vi "Main FTS.vi"() -> ()   [LabVIEW 2015]
uses:
  Controls/Gen2 FT states.ctl
  SubVI/ESTOP CONTROL.ctl
  Controls/Target RF Channel.ctl
  Controls/InfoPacket.ctl
  Controls/FTS Main Current Channel.ctl
  <vilib>/Utility/error.llb/DialogType.ctl
  Controls/LocalVars.ctl
  Controls/Iniial Device Programming.ctl
  SubVI/ProgramStageControl.ctl
  Controls/Batt Cap Steps.ctl
  Controls/Support Script.ctl
  Controls/Serial Table.ctl
  Controls/Device Information.ctl
  Controls/Loading.ctl
  Controls/Load Step.ctl
  Controls/Mark10 Config.ctl
  Controls/PID parameters.ctl
  Controls/Channels.ctl
  RxTx/XceiverStates.ctl
  Controls/Mark10 states.ctl
  RxTx/XceiverCmds.ctl
  Controls/Gen2 FT Globals.vi
  <vilib>/Utility/config.llb/Write Key (I32).vi
  <vilib>/Utility/config.llb/Write Key (String).vi
  <vilib>/Utility/config.llb/NI_LVConfig.lvlib
panel:
  out "Prog Page #":i32
  out "Time:":timestamp
  out "Transceiver Channel":u8 caption="Start Channel"
  in  "Start Channel":T1="5"
  out "Main":i32
  out "Read":i32
  in  "Correction Factor":string caption="Correction Factor:"
  out "Current Time:":timestamp=timestamp(3438190648.7035365 s since 1904-01-01) format="%<%I:%M:%S %p\n%m/%d/%Y>T"
  in  "Tab Control":T2(tab)
  in  "Eng Log?":bool
  in  "Blast Shutdown":bool=TRUE
  in  "Home":bool
  in  "GotoPosition":bool
  in  "GotoLoad":bool
  in  "Position(inch)":dbl format="%.2f"
  in  "Load(lbs):":dbl format="%.2g"
  in  "MoveUp":bool
  in  "MoveDown":bool
  in  "StopMotor":bool
  out "Gauge Load":dbl format="%.2f"
  out "Gauge Position":dbl format="%.3f"
  out "RawData":u16[](array[numeric]) caption="RawData\n      S2           S3             S4           S5           S6           S7          Ref1       Ref2        Batt"
  out "Adj.Data":dbl[](array[numeric])
  out "Front Panel Data":dbl[][](array[numeric]) format="%.2f"
  in  "Mark-10 COM Port":refnum<visa-resource-name>="COM1"
  in  "Override 4th Test":bool=TRUE
  in  "Reset Device":bool=TRUE
  out "Device Parameters":T3 {"ASICtrim" format="%02x"}
  out "GotCal":bool
  out "Streaming Serial Number":u32
  in  "Refresh Button":bool
  in  "Change Path":bool
  out "Serial Folder Path":path
  out "Serial Table Lookup":string[][](array[string]) caption="Serial Number               Lot Number            Brand Prefix              Type                        Device ID"
  in  "Close Xsceiver":bool
  in  "Scan Channels":bool
  in  "Clear Messages":bool caption="DevOFF"
  out "Test Result":bool
  in  "Operator":string caption="Operator Name:"
  in  "Target Channel":T4="5"
  in  "Operating Channel":string(combo)="5"
  out "Rev String":string
  out "Device Image":picture
  out "Battery Voltage":dbl format="%.2g"
  out "Accelerometer sample size":i32
  out "Base Accels":dbl[][](array[numeric])
  out "Six Plane Accels":dbl[][](array[numeric])
  in  "CaptureButton":bool
  out "Message":string
  out "AssemScore":i32
  out "PCB Score":i32
  out "Three Failed Tests":dbl
  out "Unit failed 3x Tests":bool
  in  "Target Serial#:":u32 caption="Serial#:" max=268435455
  out "Brand:":string
  out "DeviceType:":string
  out "Device ON?":bool
  in  "Test Device":bool
  out "SoftwareVersion":string="SW-03004-000\nRevision 1.0"
  out "DeviceID:":string
  out "Lot#:":string
  in  "ClearBuffer":bool
  in  "Exit":bool
  in  "Estop":T5
  in  "Shutdown Dev":bool caption="DevOFF"
  in  "States":T6=enum."Initialization"
  out "error out":errorcluster
  # "©2013 Aztera LLC"
  # "OrthoSensor Device Calibration"
  # "System Messages"
  # "Device"
  # "Device Information"
  # "Required Inputs"
  # "lbs"
  # "inch"
  # "Mark-10"
  # "Target Loads\n(lbs)"
  # "Gauge Loads\n(lbs)"
  # "Total Device \nLoads (lbs)"
  # "Device Loads"
  # "Errors"
  # "A (lbs)            B (lbs)"
  # "A (lbs)            B (lbs)"
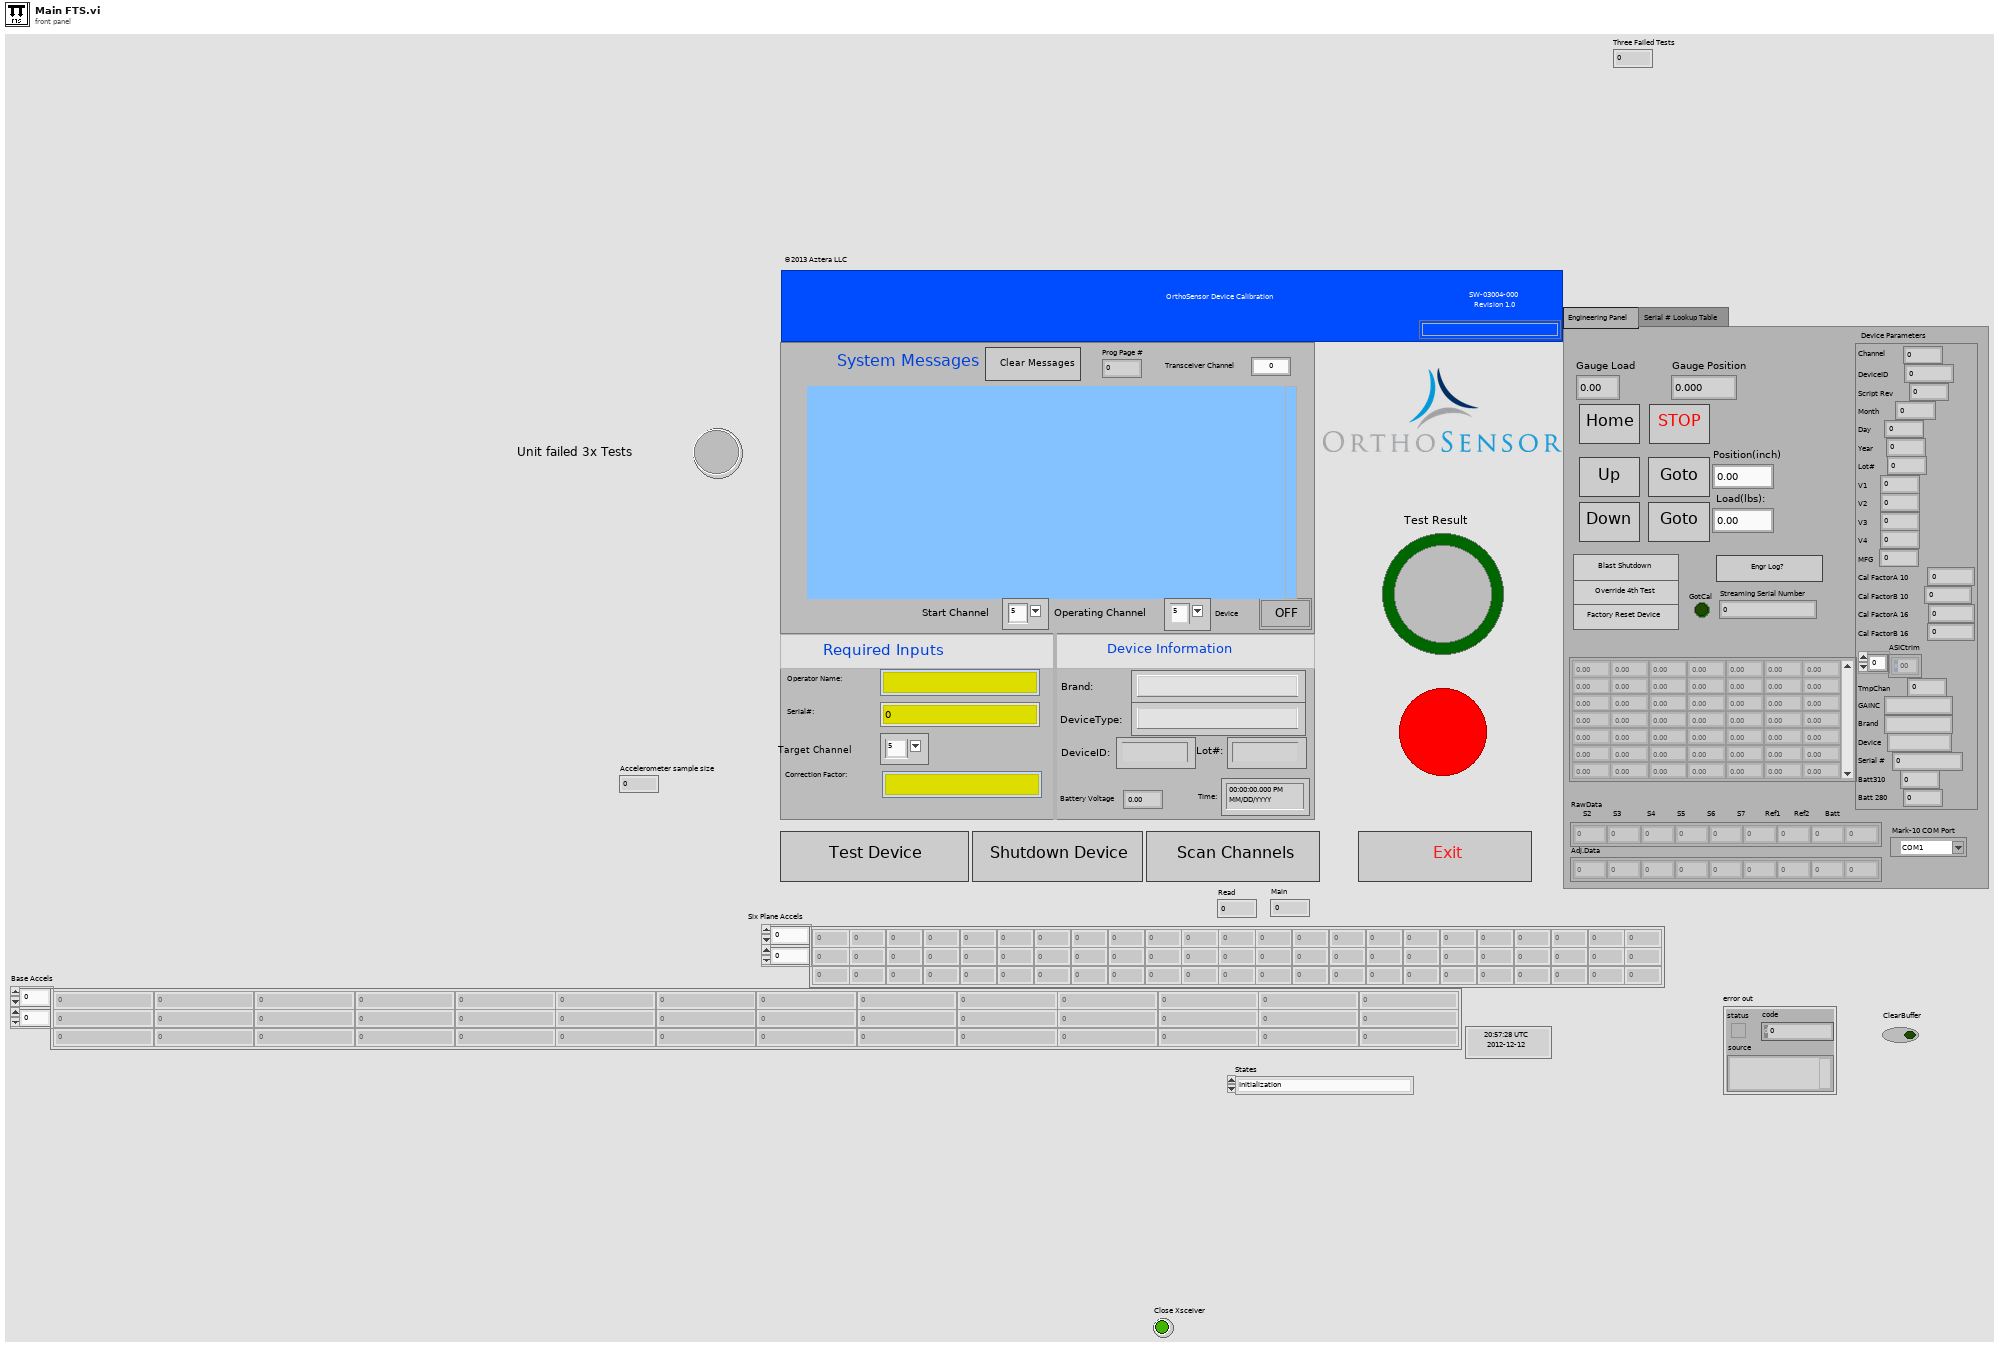
[diagram p1: front panel]
types:
  T1 = typedef "FTS Main Current Channel.ctl" = string
  T2 = enum32{"Engineering Panel", "Serial # Lookup Table"}
  T3 = typedef "InfoPacket.ctl" = cluster{"Channel":u8, "DeviceID":u32, "Script Rev":u8, "Month":u8, "Day":u8, "Year":u8, "Lot#":u32, "V1":u16, "V2":u16, "V3":u16, "V4":u16, "MFG":u8, "Cal FactorA 10":u8, "Cal FactorB 10  ":u8, "Cal FactorA 16":u8, "Cal FactorB 16":u8, "ASICtrim":u8[], "TmpChan":u8, "GAINC":string, "Brand":string, "Device":string, "Serial #":u64, "Batt310":u16, "Batt 280":u16}
  T4 = typedef "Target RF Channel.ctl" = string
  T5 = typedef "ESTOP CONTROL.ctl" = bool
  T6 = typedef "Gen2 FT states.ctl" = enum16{"---------SETUP-------", "Initialization", "Read Support Data", "Initialize Mark-10", "Initialize Transceiver", "------UTILITIES------", "Change DUT Channel", "Find RxTx Window", "Reset Device", "Scan Channels", "Read Serial Lookup", "Shutdown Device", "ESTOP", "--------USER---------", "Timeout", "-----PROGRAM-----", "Program Device", "------MARK10--------", "Go Home", "MoveUp", "MoveDown", "Goto Load", "Goto Position", "Stop Motor", "---------TESTS--------", "Start Test", "Angle Test", "Load Test", "Load Accuracy Test", "Battery Test", "------RESULTS-------", "End Test", "Display Result", "--------EXIT--------", "Exit"}
  T7 = typedef "XceiverStates.ctl" = enum16{"Initialize", "Rx", "Tx", "Raw Mode", "Clear Buffer", "ClearEcho", "Read Buffer", "Close"}
  T8 = typedef "LocalVars.ctl" = cluster{"Message":string, "Homed?":bool, "NextState":T6, "G.Load":dbl, "G.Position":dbl, "Load#":i32, "[G.Loads]":dbl[], "[TotalLoads]":dbl[], "[Errors]":dbl[][], "ZeroWait":u32, "Results":dbl[], "DwellWait":bool, "Test Result":bool, "[CondyleLoads]":dbl[][], "[Max]":dbl[], "[Min]":dbl[], "Valid String?":bool, "ScanTime":timestamp, "ScannedString":string, "LabelDevID":u32, "MfgDate":timestamp, "[EEPROM Cmds]":u8[][], "[CalData]":u8[][], "[A/Ds]":dbl[][], "[A/Dmax]":dbl[], "[A/Dmin]":dbl[], "BattMax":dbl, "BattMin":dbl, "DwellTime":i32, "PendingDeviceType":string, "Zero G.load":dbl, "GAINC Value":string, "Programming Step":T9, "Front Panel Program?":bool, "Final Program?":bool, "PCB Score":i32, "AssyScore":i32, "Pass/Fail #":string, "Result String":string, "Programming Mode":T10, "Angle Test Step":enum16{"Initialize", "Get X", "Get Y", "Get Z", "Next Test"}, "Accel Values":dbl[][], "Shutdown Counter":u32, "V1":i32, "V2":i32, "V3":i32, "V4":i32, "EEPROM Data":i32[][], "Counter":i32, "Page#":i32, "Timer":timestamp, "Use Mark10?":bool, "Eng-Result#":u32, "DUT Serial #":i32, "Scroll Message?":bool, "Clear Message":bool, "Batt Test Step ":T11, "RXTX Window Found?":bool, "Shutdown First Call?":bool, "A2 Delay (msec)":i16, "Support Script":T12, "Serial Table":T13, "Target Information":T14, "Operator":string, "COM Port":string, "Config Path":path, "Tx Array":u8[], "DUT Parameters":T3, "FTS Main?":bool, "Loading":T15, "Software Version":string, "Correction Factor":string, "Second Load Test":bool, "Acc Loads":dbl[][], "Mark10 Config":T17, "Channels":T19, "Channel EEPROM":i32[][], "Load Notes":string[], "Engr Log?":bool, "Time":timestamp[], "Program Retry":bool, "Operator Channel":string, "Target Channel ":string, "New Data Program":bool, "NFHU Pass?":bool, "Cycle Number":i32, "Cal Cycle#":i32, "[Avg G.Loads] ":dbl[], "[Avg A/Ds] ":dbl[][], "Cal Retry?":bool, "[Total A/Ds]  ":dbl[][], "Cycle Num LA":i32, "LA Cycle# ":i32, "Shim Num":i32, "Shim#  ":i32, "Angle Test?":bool}
  T9 = typedef "Iniial Device Programming.ctl" = enum16{"Load EEPROM", "Send First A1", "Send EEPROM", "Send A1", "Check EEPROM Echo", "Verify transmission", "Programming Successful", "Programming Failed"}
  T10 = typedef "ProgramStageControl.ctl" = enum16{"Initial Program", "GainC", "Scales"}
  T11 = typedef "Batt Cap Steps.ctl" = enum16{"Initialize", "Collect 2.8 Volts", "Collect 3.1 Volts", "Check Results"}
  T12 = typedef "Support Script.ctl" = cluster{"Script #":string, "Script Revision":string, "[OEMs]":string[], "[[DeviceTypes]]":string[][], "[[DeviceTypesVals]]":u16[][], "[[List of Errors]]":string[][], "Default GAINC":string, "[[ASICtrims]]":u8[][], "ID For Echo":string, "Condyle A CalFactor":i32, "Condyle B CalFactor":i32, "[OEMs Prefix]":string[], "Packet ID 18":string, "[[Force Table Load Test]]":dbl[][], "[[Force Table AccurTest]]":dbl[][]}
  T13 = typedef "Serial Table.ctl" = cluster{"Serial File Path":path, "[[Serial Lookup Table]]":string[][], "Serial Device Info":string[], "Valid Serial?":bool}
  T14 = typedef "Device Information.ctl" = cluster{"Target Brand":string, "Target DeviceType":string, "Target Serial#":i32, "Target Lot#":u32, "Target DevID":u32, "Target Channel":u8}
  T15 = typedef "Loading.ctl" = cluster{"[Forces]":dbl[], "[Dwell]":dbl[], "Loading Step":T16}
  T16 = typedef "Load Step.ctl" = enum16{"Initialize Test", "Go Home", "Detect Dev Surface", "Wait to zero Device", "Zero Device", "Do Test", "Test Result"}
  T17 = typedef "Mark10 Config.ctl" = cluster{"H2S%":dbl[], "H2S Speed":dbl[], "H to S":dbl, "Home Speed":dbl, "LoadWin":dbl, "Load Speed":dbl, "PID":T18}
  T18 = typedef "PID parameters.ctl" = cluster{"Kp":dbl, "Kd":dbl, "Ki":dbl}
  T19 = typedef "Channels.ctl" = cluster{"Transceiver Ch":u8, "Operating Ch":u8, "Start Ch":u8}
  T20 = typedef "DialogType.ctl" = u16
  T21 = enum8{"Enabled", "Disabled", "Disabled and Grayed Out"}
  T22 = enum16{"None", "On Hover", "On Key Focus", "On Hover or Key Focus"}
  T23 = typedef "Mark10 states.ctl" = enum16{"Initialize", "Go Home", "Move Up", "Move Down", "Stop @ Load", "Read Status", "Goto Position", "Goto Device Surface", "Stop Motor", "Shutdown", "Exit"}
  T24 = typedef "XceiverCmds.ctl" = enum8{"Get Window", "Set Window", "Load&Xmit", "Find Window", "Load CC1101", "Blink LED1", "Blink LED2", "Gen2 Mode", "Request Rev", "Gen2 Mode & Req Rev", "Load Device Settings", "Reset Xceiver", "Set Channel", "Read Channel"}
  T25 = cluster{"Shift":bool, "Ctrl":bool, "Alt":bool, "Cmd":bool, "Opt":bool}
  T26 = typedef "Scanned Data.ctl" = cluster{"DeviceID":u32, "Mfg Date":timestamp, "ScannedIn":bool, "Lot#":u32}
  T27 = typedef "LVRectTypeDef.ctl" = cluster{"Left":i16, "Top":i16, "Right":i16, "Bottom":i16}
  T28 = typedef "NI_LVConfig.lvlib/Config Data RefNum.ctl" = refnum<k1>
  T29 = typedef "DeviceInfo.ctl" = cluster{"DevInfo":T3, "Mfg Date":timestamp, "[CalData]":u8[][], "[DevData]":u8[], "GotCal":bool, "CustomCal?":bool, "Packet#":i32}
  T30 = enum16{"Initialize", "Get X", "Get Y", "Get Z", "Next Test"}
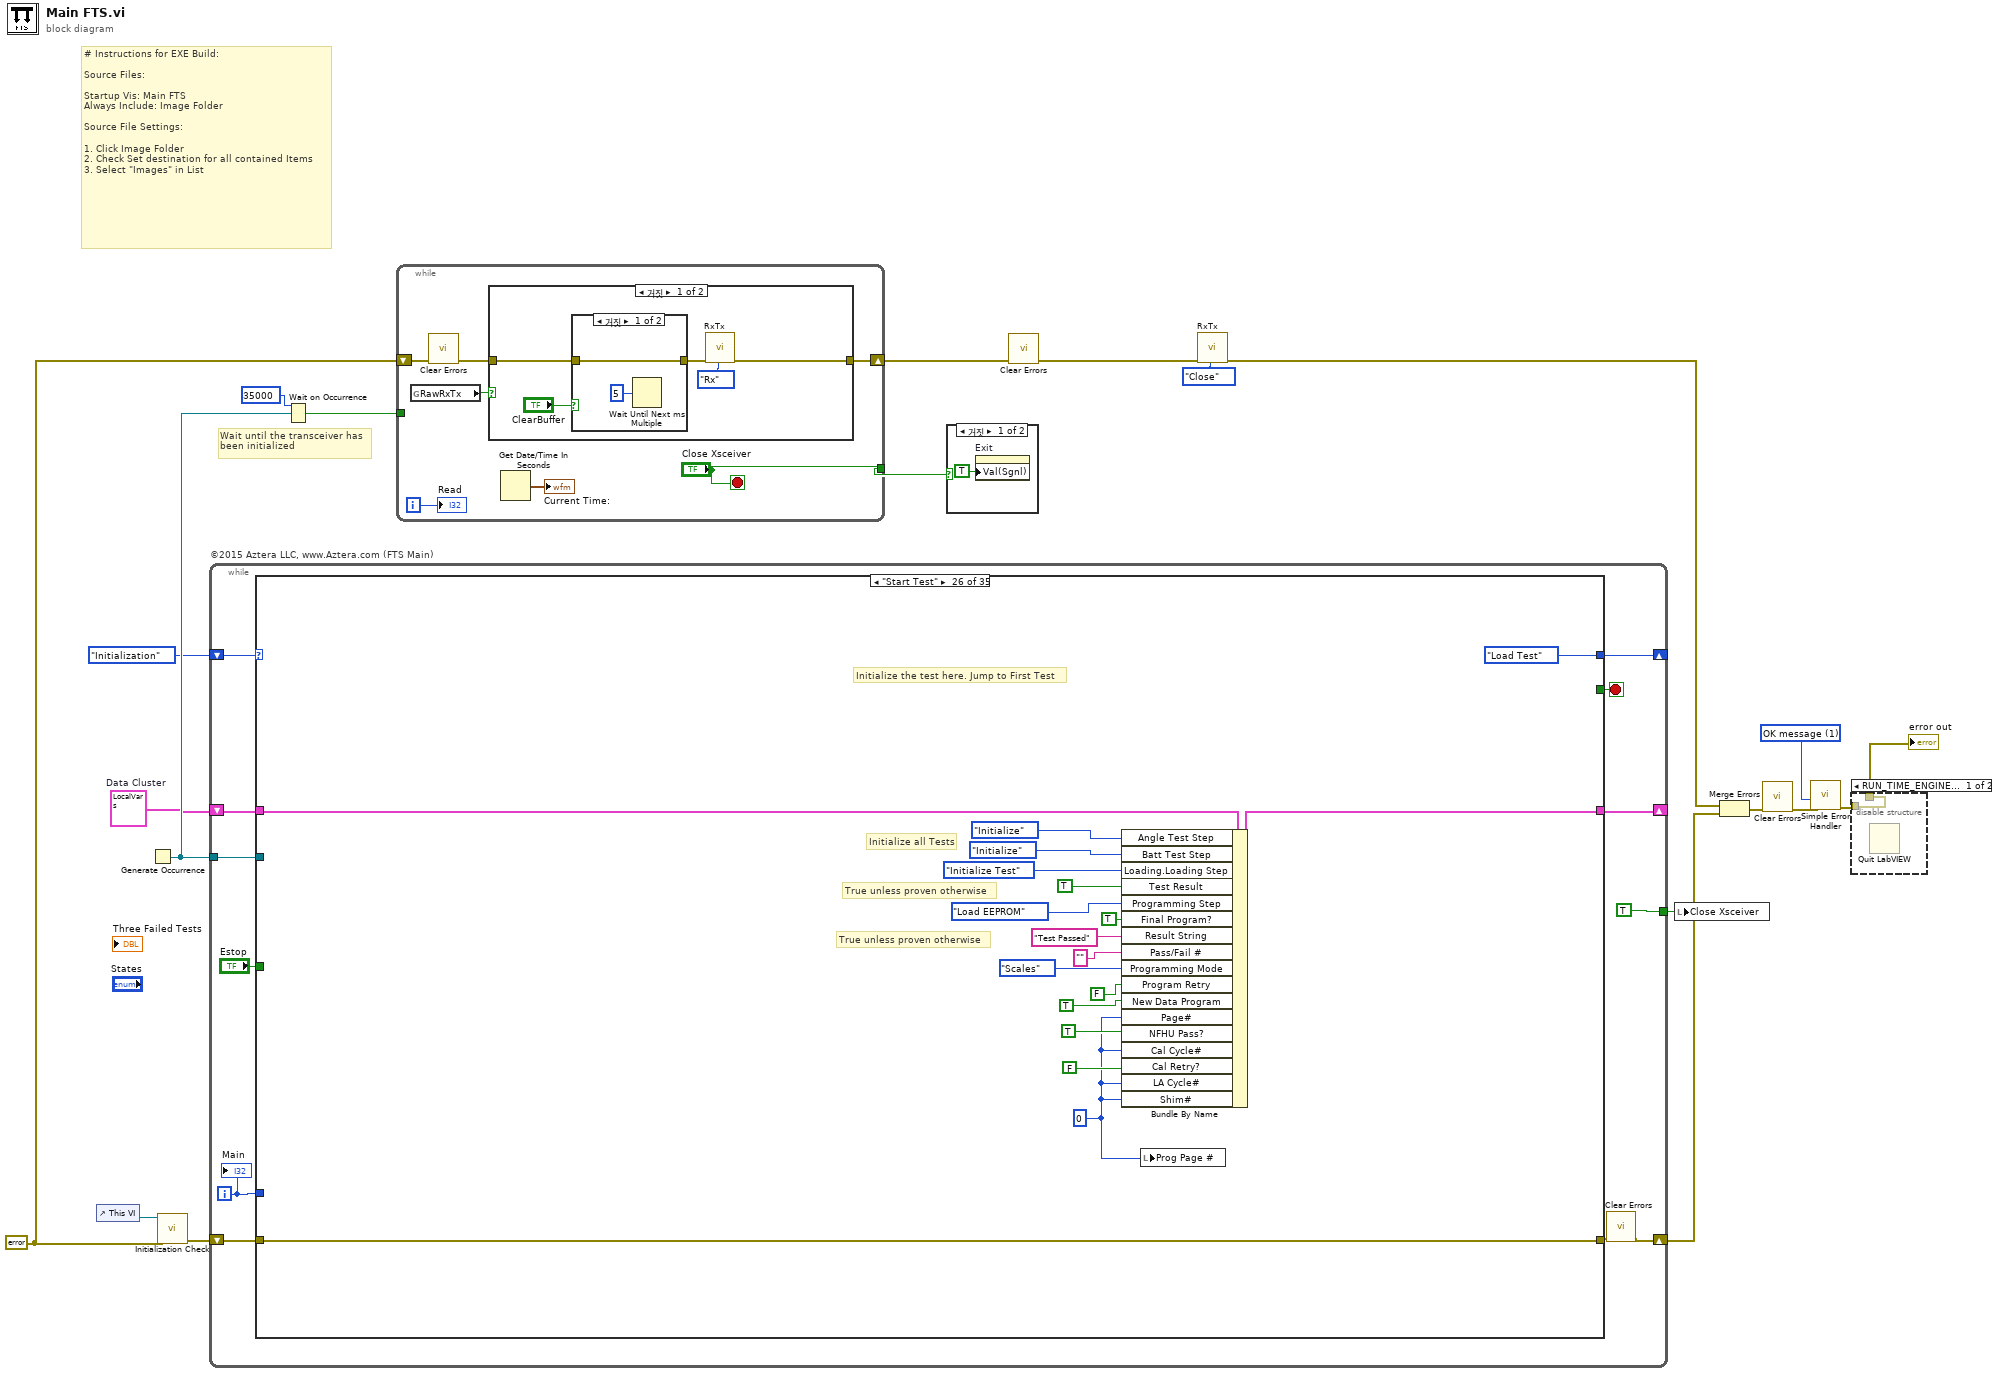
[diagram p0: block diagram]
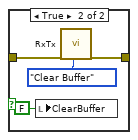
[diagram p2: hidden frame]
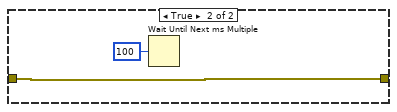
[diagram p3: hidden frame]
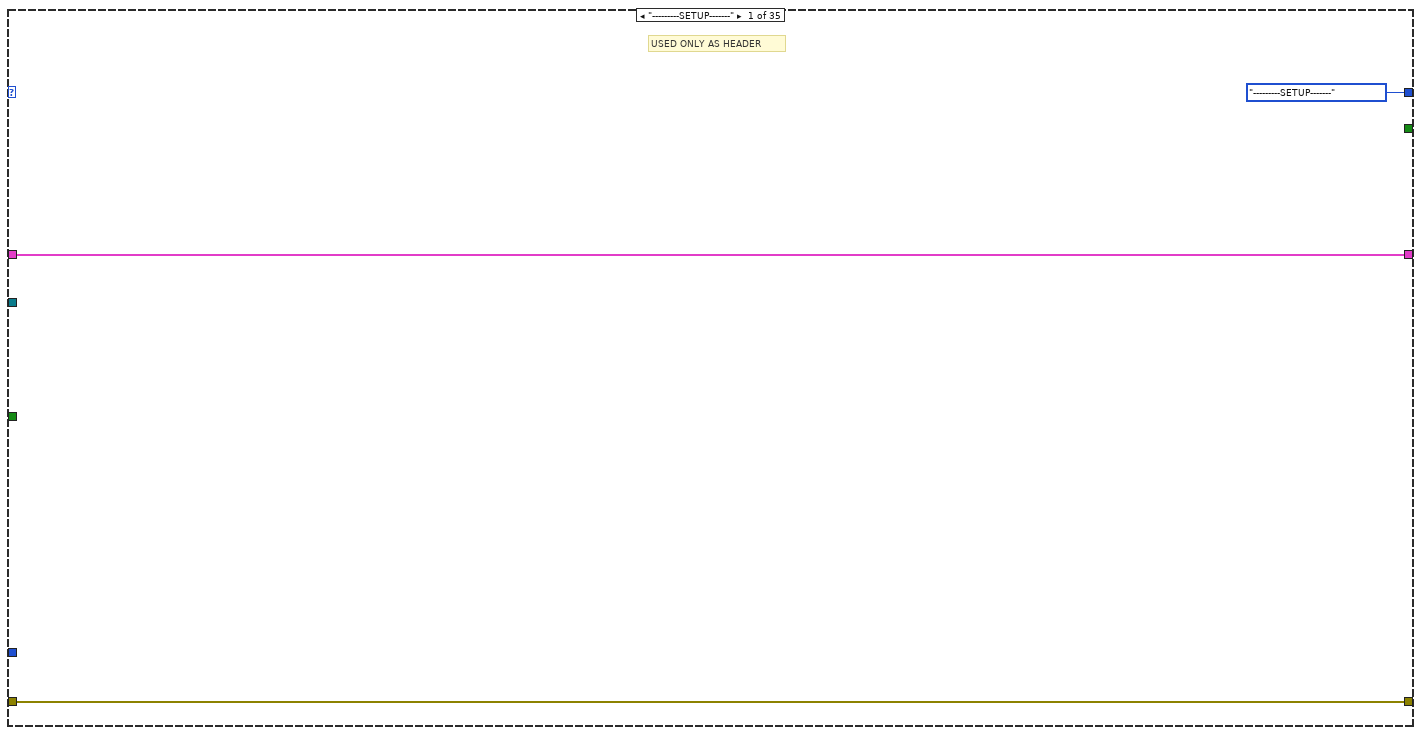
[diagram p6: hidden frame]
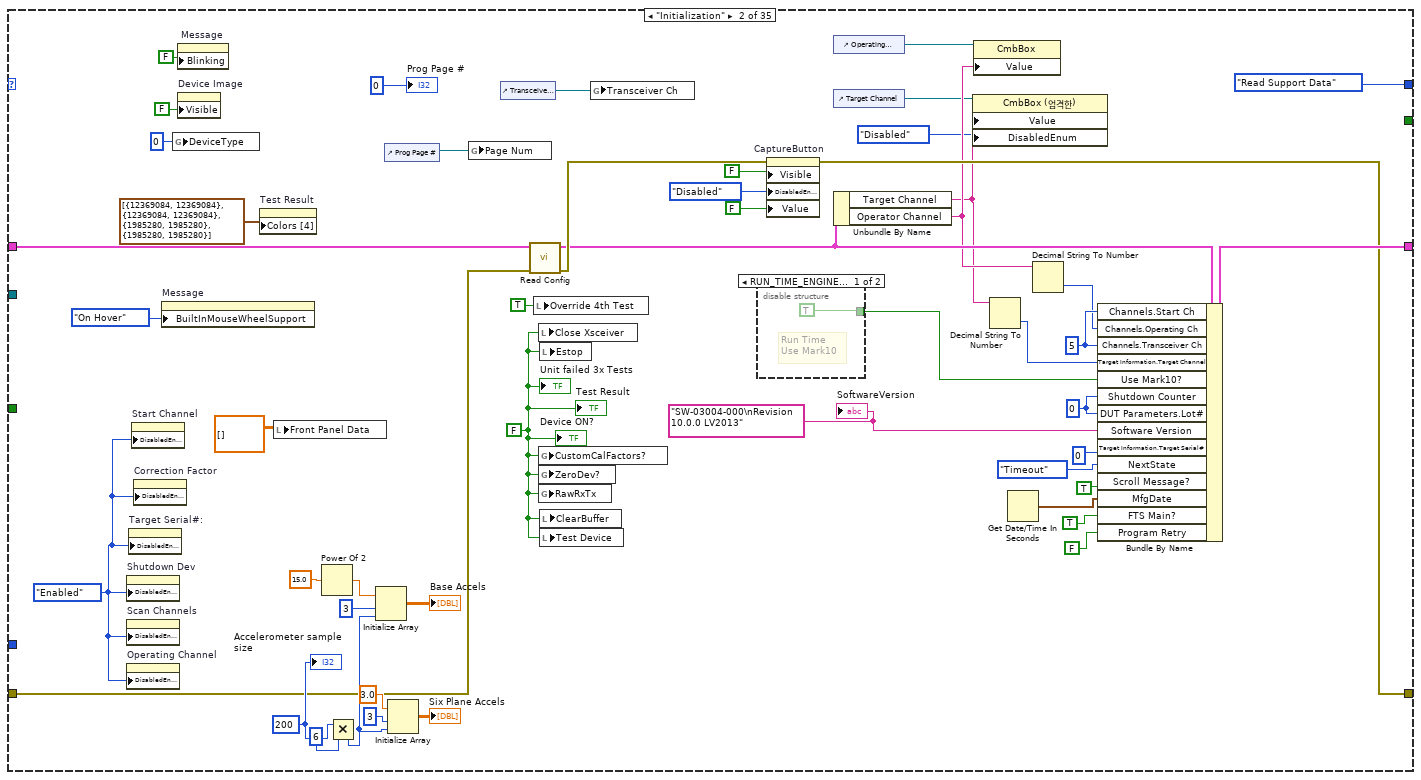
[diagram p7: hidden frame]
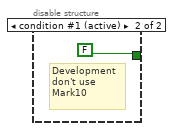
[diagram p8: hidden frame]
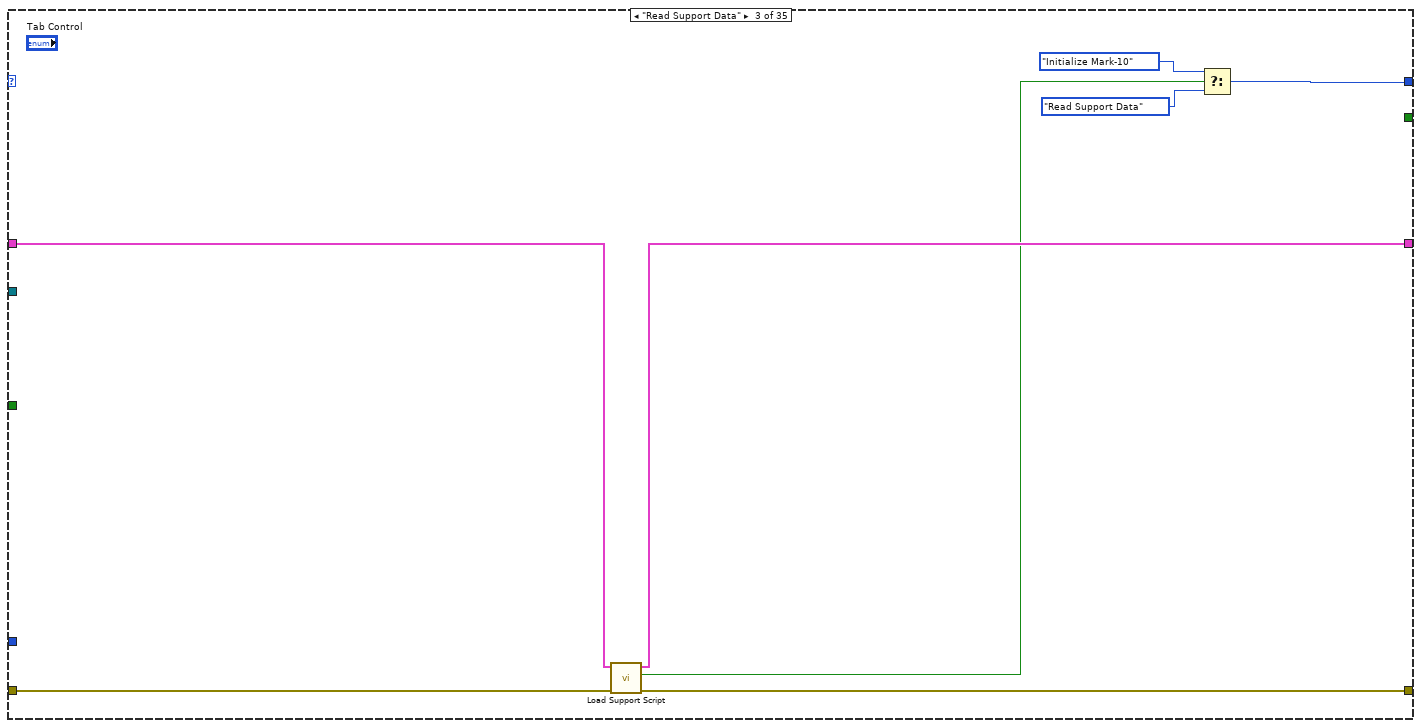
[diagram p9: hidden frame]
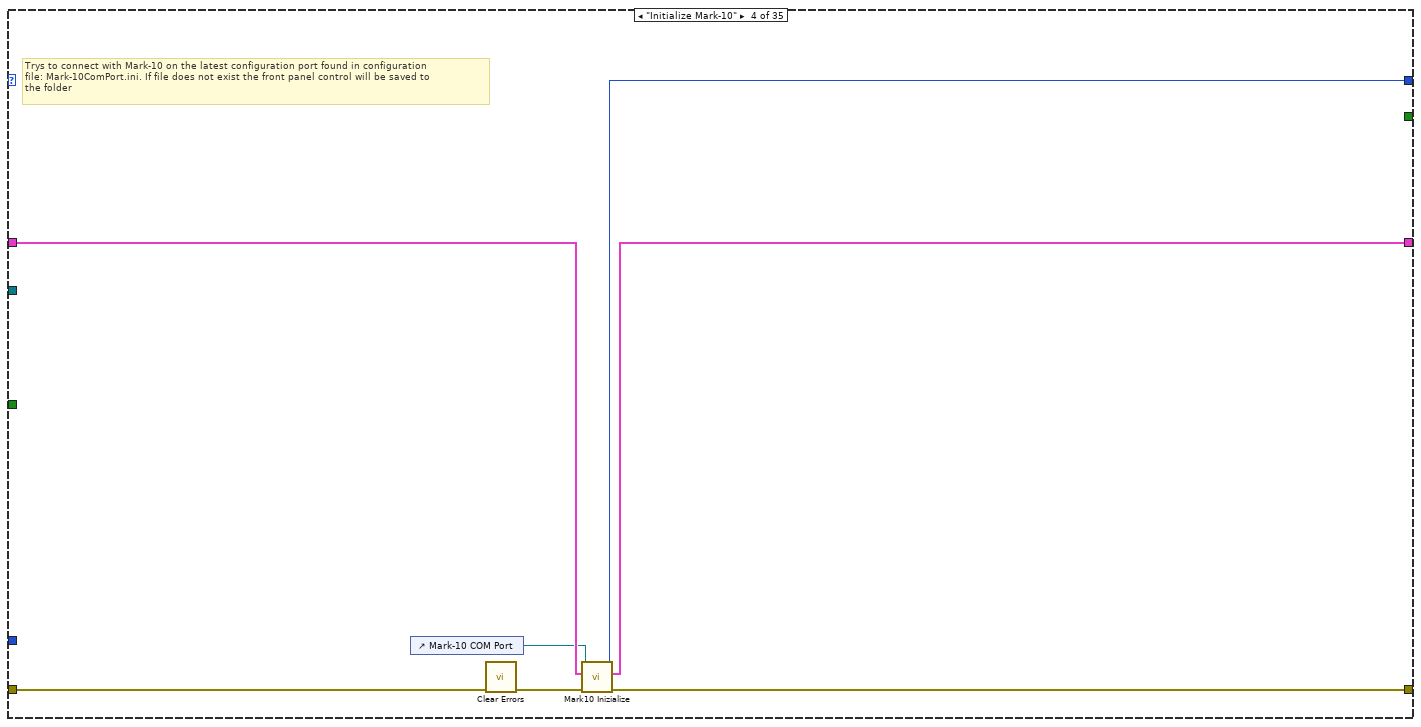
[diagram p10: hidden frame]
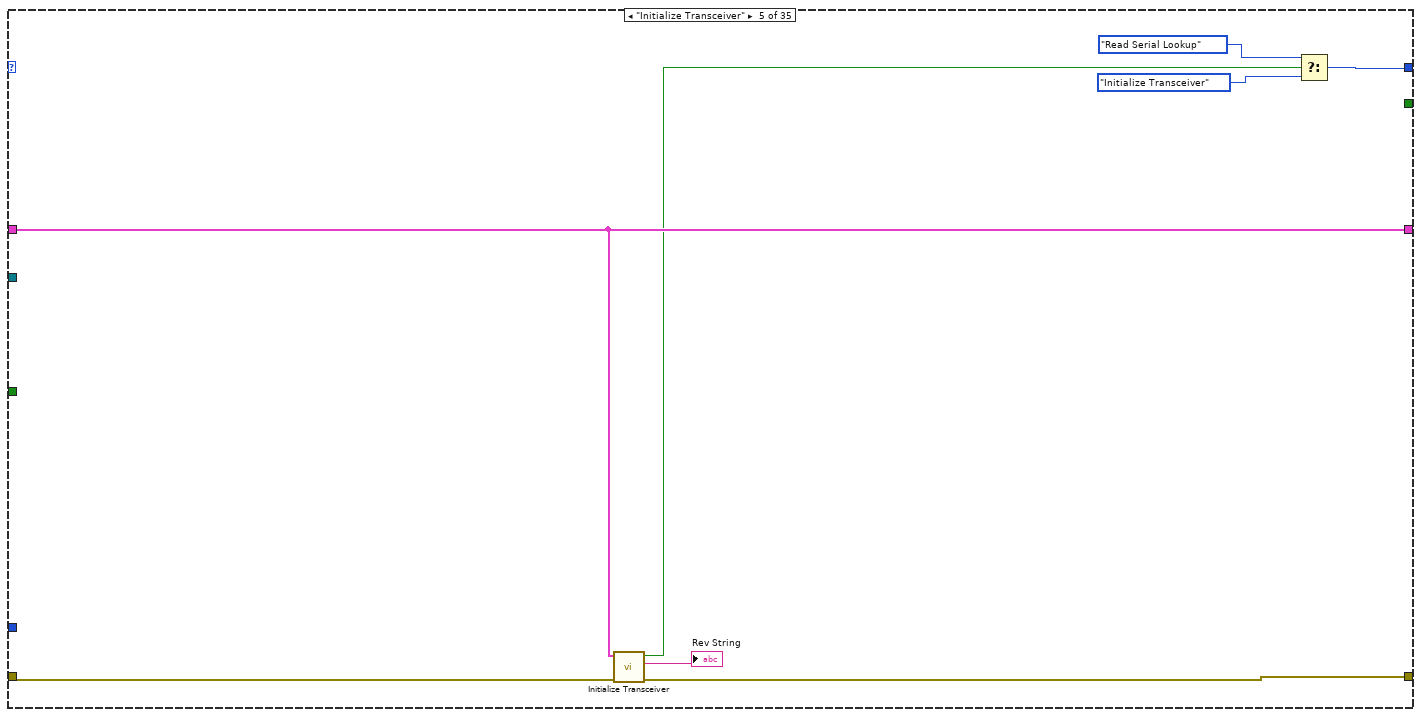
[diagram p11: hidden frame]
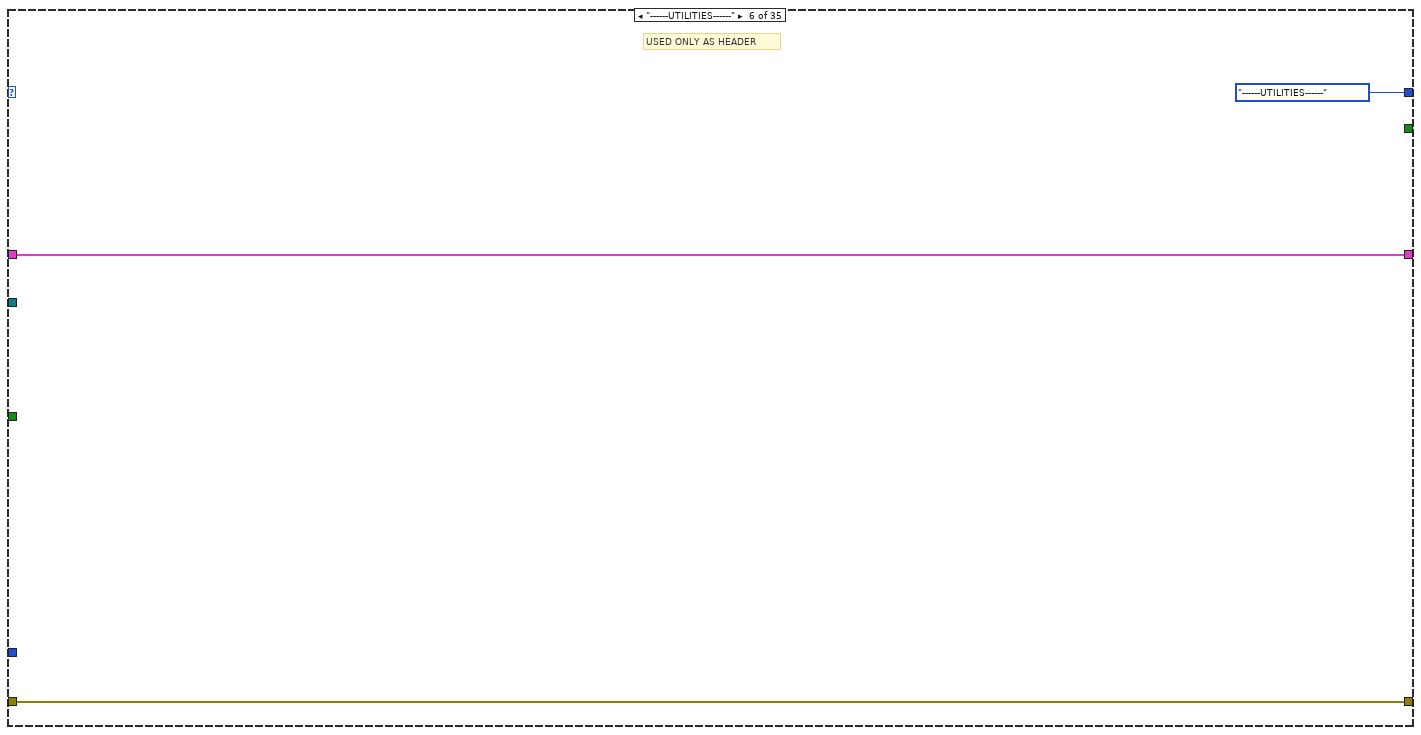
[diagram p12: hidden frame]
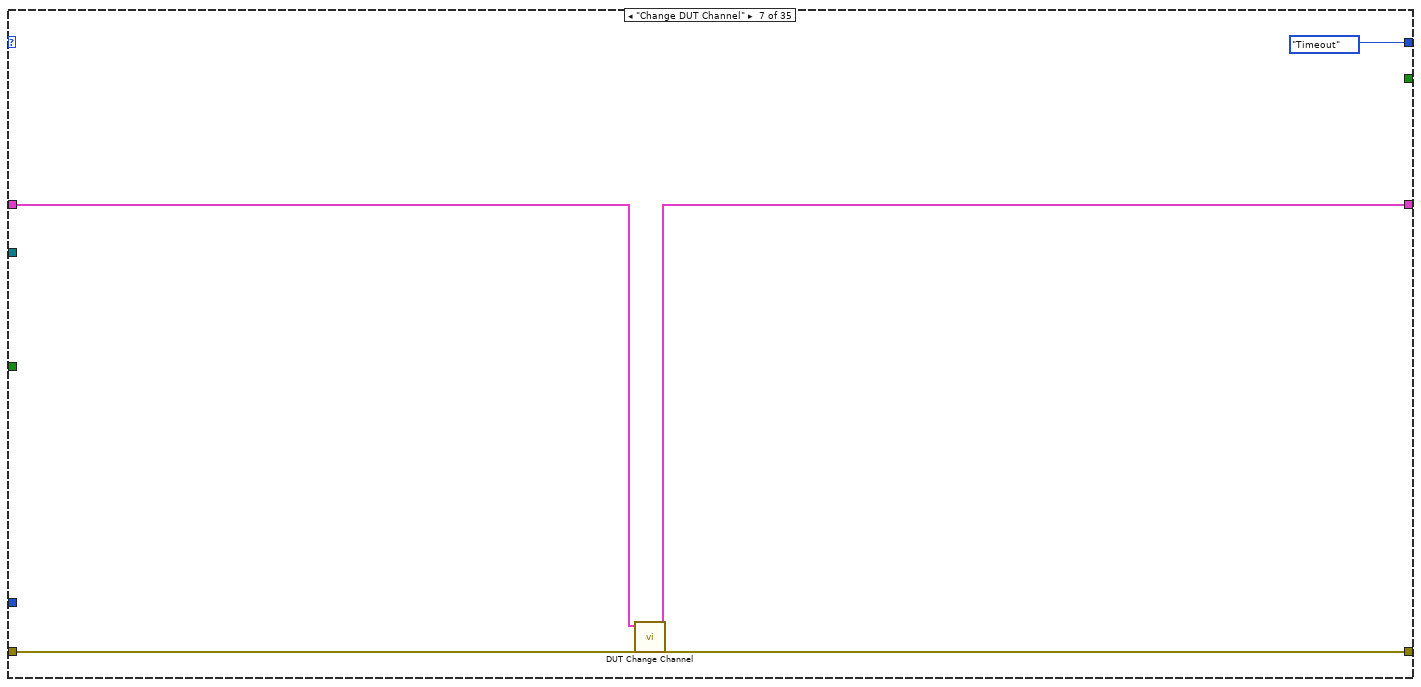
[diagram p13: hidden frame]
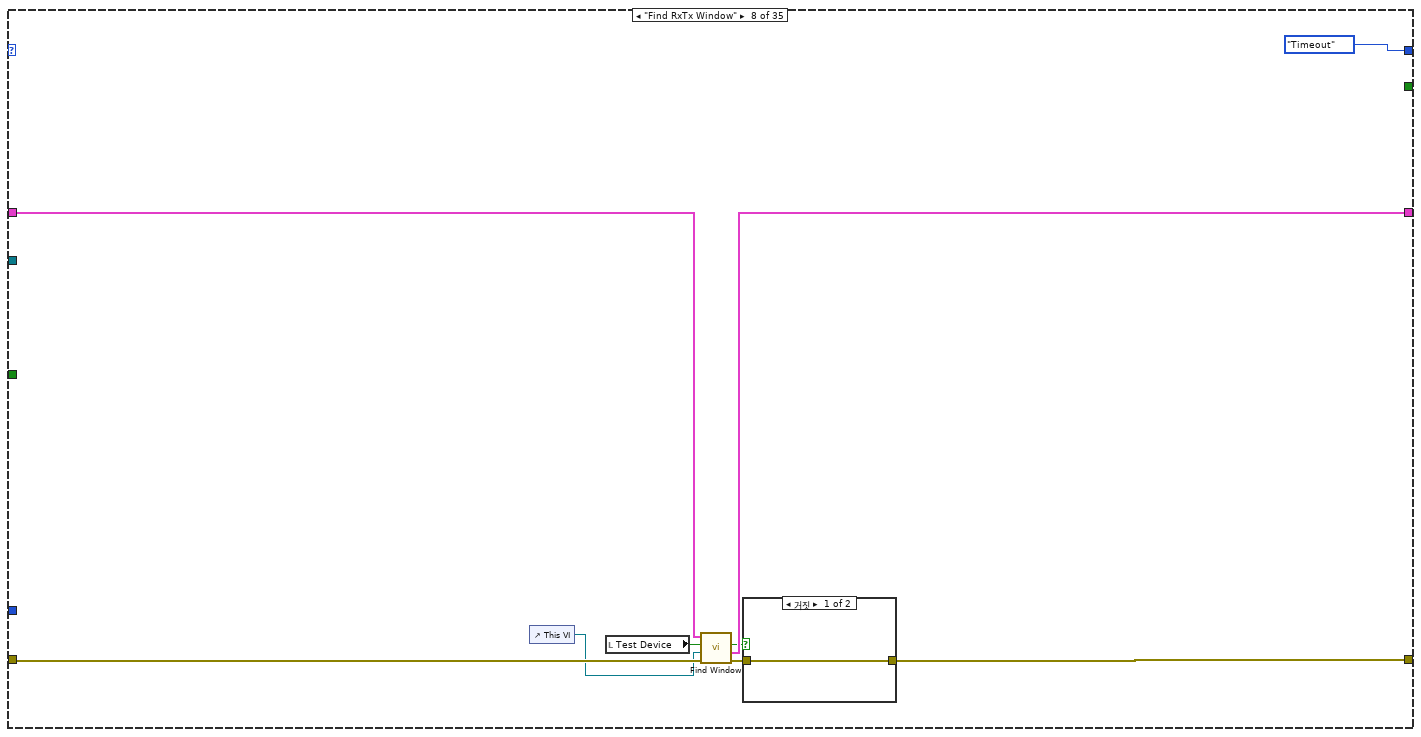
[diagram p14: hidden frame]
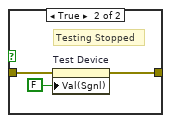
[diagram p15: hidden frame]
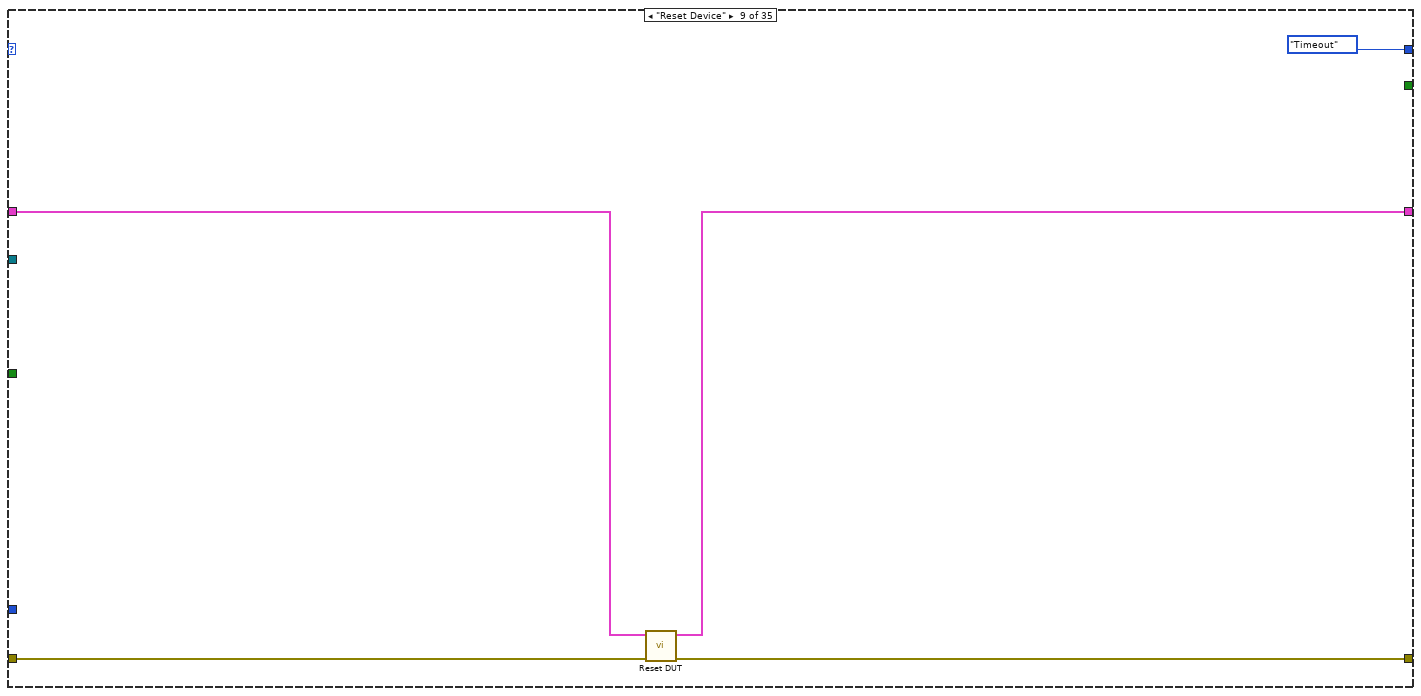
[diagram p16: hidden frame]
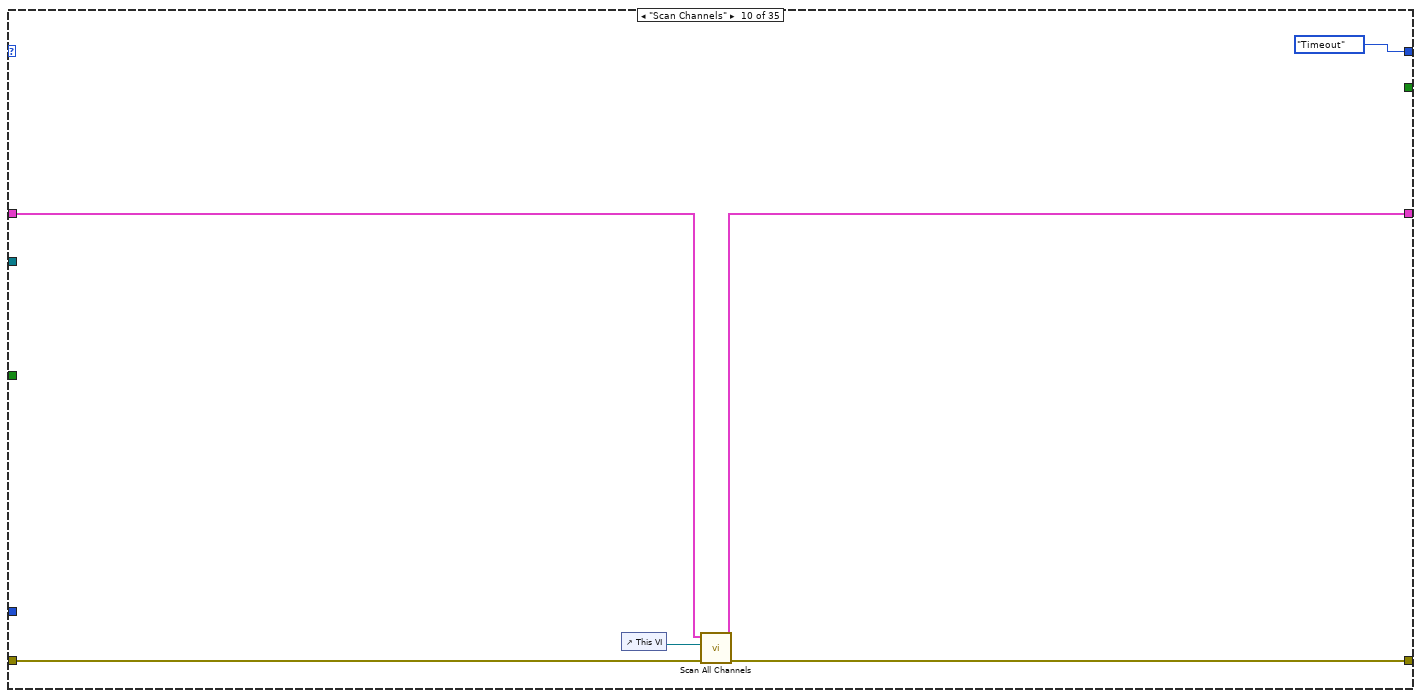
[diagram p17: hidden frame]
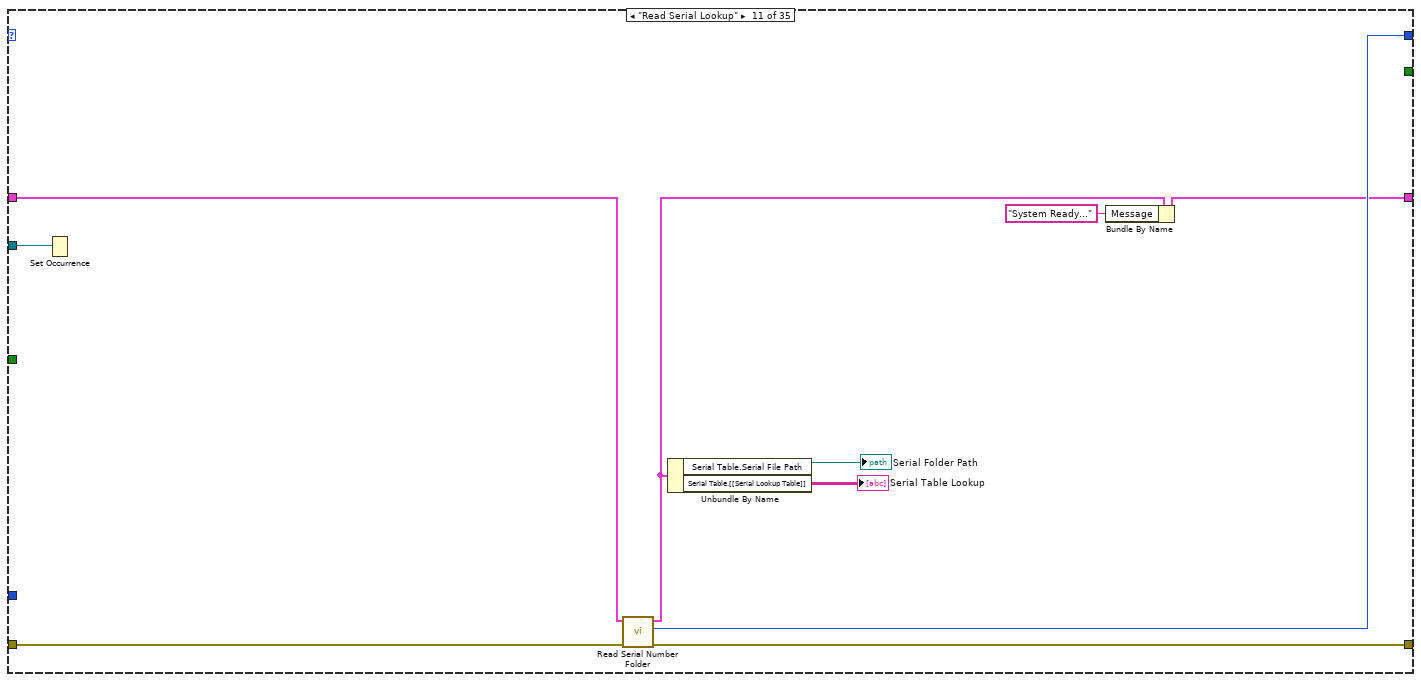
[diagram p18: hidden frame]
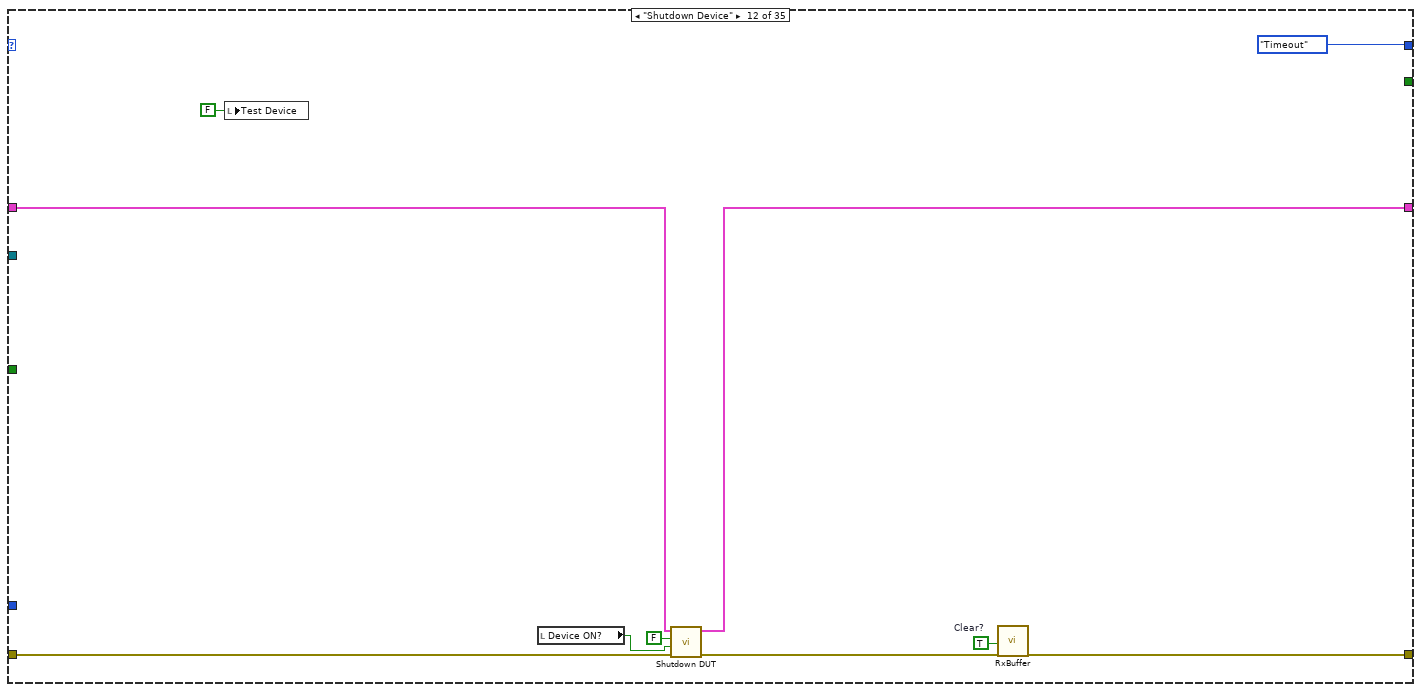
[diagram p19: hidden frame]
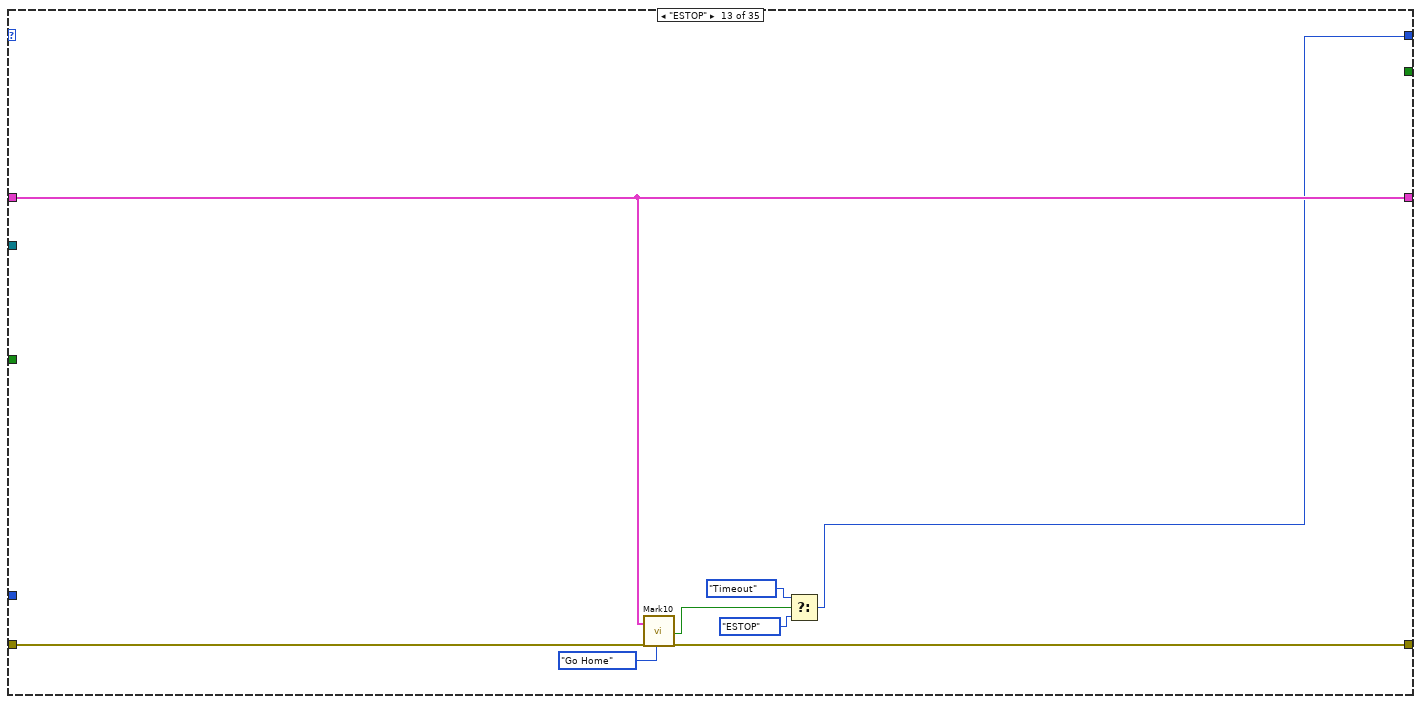
[diagram p20: hidden frame]
diagram:
  w4 = errorcluster {"status"=FALSE, "code"=0, "source"=""} ("error in (no error)")
  w10 = T8 {"Message"="", "Homed?"=FALSE, "NextState"=enum."Scan Channels", "G.Load"=0.0, "G.Position"=0.0, "Load#"=0, "[G.Loads]"=[], "[TotalLoads]"=[], "[Errors]"=[], "ZeroWait"=0, "Results"=[], "DwellWait"=FALSE, "Test Result"=FALSE, "[CondyleLoads]"=[], "[Max]"=[], "[Min]"=[], "Valid String?"=FALSE, "ScanTime"=timestamp(0 s since 1904-01-01), "ScannedString"="", "LabelDevID"=0, "MfgDate"=timestamp(0 s since 1904-01-01), "[EEPROM Cmds]"=[], "[CalData]"=[], "[A/Ds]"=[], "[A/Dmax]"=[], "[A/Dmin]"=[], "BattMax"=0.0, "BattMin"=0.0, "DwellTime"=0, "PendingDeviceType"="", "Zero G.load"=0.0, "GAINC Value"="", "Programming Step"=enum."Load EEPROM", "Front Panel Program?"=FALSE, "Final Program?"=FALSE, "PCB Score"=0, "AssyScore"=0, "Pass/Fail #"="", "Result String"="", "Programming Mode"=enum."Initial Program", "Angle Test Step"=enum."Initialize", "Accel Values"=[], "Shutdown Counter"=0, "V1"=0, "V2"=0, "V3"=0, "V4"=0, "EEPROM Data"=[], "Counter"=0, "Page#"=0, "Timer"=timestamp(0 s since 1904-01-01), "Use Mark10?"=FALSE, "Eng-Result#"=0, "DUT Serial #"=0, "Scroll Message?"=FALSE, "Clear Message"=FALSE, "Batt Test Step "=enum."Initialize", "RXTX Window Found?"=FALSE, "Shutdown First Call?"=FALSE, "A2 Delay (msec)"=0, "Support Script"={"Script #"="", "Script Revision"="", "[OEMs]"=[], "[[DeviceTypes]]"=[], "[[DeviceTypesVals]]"=[], "[[List of Errors]]"=[], "Default GAINC"="", "[[ASICtrims]]"=[], "ID For Echo"="", "Condyle A CalFactor"=0, "Condyle B CalFactor"=0, "[OEMs Prefix]"=[], "Packet ID 18"="", "[[Force Table Load Test]]"=[], "[[Force Table AccurTest]]"=[]}, "Serial Table"={"Serial File Path"=path "", "[[Serial Lookup Table]]"=[], "Serial Device Info"=[], "Valid Serial?"=FALSE}, "Target Information"={"Target Brand"="", "Target DeviceType"="", "Target Serial#"=0, "Target Lot#"=0, "Target DevID"=0, "Target Channel"=0}, "Operator"="", "COM Port"="", "Config Path"=path "", "Tx Array"=[], "DUT Parameters"={"Channel"=0, "DeviceID"=0, "Script Rev"=0, "Month"=0, "Day"=0, "Year"=0, "Lot#"=0, "V1"=0, "V2"=0, "V3"=0, "V4"=0, "MFG"=0, "Cal FactorA 10"=0, "Cal FactorB 10  "=0, "Cal FactorA 16"=0, "Cal FactorB 16"=0, "ASICtrim"=[], "TmpChan"=0, "GAINC"="", "Brand"="", "Device"="", "Serial #"=0, "Batt310"=0, "Batt 280"=0}, "FTS Main?"=FALSE, "Loading"={"[Forces]"=[], "[Dwell]"=[], "Loading Step"=enum."Initialize Test"}, "Software Version"="", "Correction Factor"="", "Second Load Test"=FALSE, "Acc Loads"=[], "Mark10 Config"={"H2S%"=[], "H2S Speed"=[], "H to S"=0.0, "Home Speed"=0.0, "LoadWin"=0.0, "Load Speed"=0.0, "PID"={"Kp"=0.0, "Kd"=0.0, "Ki"=0.0}}, "Channels"={"Transceiver Ch"=0, "Operating Ch"=0, "Start Ch"=0}, "Channel EEPROM"=[], "Load Notes"=[], "Engr Log?"=FALSE, "Time"=[], "Program Retry"=FALSE, "Operator Channel"="", "Target Channel "="", "New Data Program"=FALSE, "NFHU Pass?"=FALSE, "Cycle Number"=0, "Cal Cycle#"=0, "[Avg G.Loads] "=[], "[Avg A/Ds] "=[], "Cal Retry?"=FALSE, "[Total A/Ds]  "=[], "Cycle Num LA"=0, "LA Cycle# "=0, "Shim Num"=0, "Shim#  "=0, "Angle Test?"=FALSE}  # Data Cluster
  w14 = T20 1 items=["no dialog", "OK message", "continue or stop message", "OK message + warnings", "continue/stop + warnings"] ("type of dialog (OK msg:1)")
  # "Wait until the transceiver has\nbeen initialized"
  # "# Instructions for EXE Build:\n\nSource Files:\n\nStartup Vis: Main FTS\nAlways Include: Image Folder\n\nSource File Settings:\n\n1. Click Image Folder\n2. Check Set destination for all contained Items\n3. Select \"Images\" in List"
  n1 = control-ref of="This VI"() -> (w9:refnum<vi>)
  n2 = Generate Occurrence() -> (w19:refnum<k4>)
  n3 = call "Initialization Check.vi"("error in (no error)"=w4, "VI in"=w9) -> ("error out"=w8:errorcluster)  [unwired: 9 in]
  n4 = while "©2015 Aztera LLC, www.Aztera.com (FTS Main)" {
    shift-right: [w26] -> _
    shift-left: w10 -> [w30]
    shift-right: [w27] -> w20
    shift-left: w8 -> [w31]
    tunnel: w19 -> [w24]
    tunnel: [TRUE ("Close Xsceiver")] -> w7
    shift-right: [w23] -> _
    shift-left: Gen2_FT_states."Initialization" ("Current State Out") -> [w22]
    i -> [w29]
    stop <- w21 stop-if-true
    n5 = case shown="\"Start Test\"" w22 {
      tunnel: [w35 w54 w92 w101 w108 w112 w115 w120 w132 w139 w146 w152 w167 w172 w175 w646 w648 w654 w668 w682 w709 w733 w758 w782 w786 w792 w809 w815 w818 w826 w832 w843 w879 w909 w920] -> w32
      tunnel: w31 -> [w35 w57 w94 w100 w109 w112 w116 w123 w133 w140 w150 w155 w168 w172 w176 w646 w651 w654 w669 w683 w710 w734 w759 w783 w786 w792 w809 w817 w824 w828 w832 w845 w892 w909 w914]
      tunnel: [w34 w66 w91 w98 w105 w111 w113 w125 w134 w141 w144 w158 w163 w171 w177 w645 w647 w653 w667 w681 w708 w732 w757 w776 w785 w795 w807 w816 w822 w825 w831 w849 w893 w908 w922] -> w26
      tunnel: w30 -> [w34 w58 w93 w99 w105 w111 w114 w126 w135 w137 w151 w160 w163 w171 w180 w645 w650 w653 w659 w673 w701 w728 w752 w777 w785 w793 w808 w813 w823 w829 w831 w834 w870 w908 w912]
      tunnel: w29 -> [_ _ _ _ _ _ _ _ _ _ _ _ _ _ w179 _ _ _ _ _ _ _ _ _ _ _ _ _ _ _ _ _ _ _ _]
      tunnel: "Estop" -> [_ _ _ _ _ _ _ _ _ _ _ _ _ _ w178 _ _ _ _ w676 w703 w726 w750 _ _ _ _ _ _ _ _ _ _ _ _]
      tunnel: w24 -> [_ _ _ _ _ _ _ _ _ _ w142 _ _ _ _ _ _ _ _ _ _ _ _ _ _ _ _ _ _ _ _ _ _ _ _]
      tunnel: [Gen2_FT_states."---------SETUP-------" ("Current State Out") Gen2_FT_states."Read Support Data" ("t") w88 w95 w102 Gen2_FT_states."------UTILITIES------" ("Current State Out") Gen2_FT_states."Timeout" ("Current State Out") Gen2_FT_states."Timeout" ("Current State Out") Gen2_FT_states."Timeout" ("Current State Out") Gen2_FT_states."Timeout" ("Current State Out") w145 Gen2_FT_states."Timeout" ("Current State Out") w162 Gen2_FT_states."--------USER---------" ("Current State Out") w174 Gen2_FT_states."-----PROGRAM-----" ("Current State Out") Gen2_FT_states."Timeout" ("Current State Out") Gen2_FT_states."------MARK10--------" ("Current State Out") w655 w670 w697 Gen2_FT_states."Timeout" ("Current State Out") Gen2_FT_states."Timeout" ("Current State Out") w775 Gen2_FT_states."---------TESTS--------" ("Current State Out") Gen2_FT_states."Load Test" ("Current State Out") Gen2_FT_states."Timeout" ("Current State Out") Gen2_FT_states."Timeout" ("Current State Out") Gen2_FT_states."Timeout" ("Current State Out") Gen2_FT_states."Timeout" ("Current State Out") Gen2_FT_states."------RESULTS-------" ("Current State Out") Gen2_FT_states."Timeout" ("Current State Out") Gen2_FT_states."Timeout" ("Current State Out") Gen2_FT_states."--------EXIT--------" ("Current State Out") Gen2_FT_states."Exit" ("Current State Out")] -> w23
      tunnel: [_ _ _ _ _ _ _ _ _ _ _ _ _ _ _ _ _ _ _ _ _ _ _ _ _ _ _ _ _ _ _ _ _ _ TRUE] -> w21
      frame "---------SETUP-------" {
        # "USED ONLY AS HEADER"
      }
      frame "Initialization" {
        w48 = u8 5 ("Current Channel")
        w49 = T21."Enabled" ("Disabled")
        w65 = u32 0 ("Shutdown Counter")
        w69 = 200
        w64 = "SW-03004-000\nRevision 10.0.0 LV2013" ("SoftwareVersion")
        w51 = FALSE ("Exit")
        n6 = property on="Shutdown Dev" class="Bool"("DisabledEnum"=w49) -> ()  [unwired: 2 in, 2 out]
        n7 = property on="Scan Channels" class="Bool"("DisabledEnum"=w49) -> ()  [unwired: 2 in, 2 out]
        n8 = property on="Operating Channel" class="CmbBox"("DisabledEnum"=w49) -> ()  [unwired: 2 in, 2 out]
        n9 = property on="Target Serial#:" class="DigNum (엄격한)"("DisabledEnum"=w49) -> ()  [unwired: 2 in, 2 out]
        n10 = property on="Start Channel" class="CmbBox (엄격한)"("DisabledEnum"=w49) -> ()  [unwired: 2 in, 2 out]
        n11 = property on="Correction Factor" class="Str"("DisabledEnum"=w49) -> ()  [unwired: 2 in, 2 out]
        n12 = property on="Message" class="Str"("BuiltInMouseWheelSupport"=T22."On Hover" ("Built-In Mouse Wheel Support")) -> ()  [unwired: 2 in, 2 out]
        n13 = global write "Gen2 FT Globals.vi" "DeviceType"(u32 0 ("Lot Number")) -> ()
        n14 = property on="Message" class="Str"("Blinking"=FALSE) -> ()  [unwired: 2 in, 2 out]
        n15 = property on="Device Image" class="Pict"("Visible"=FALSE) -> ()  [unwired: 2 in, 2 out]
        n16 = property on="Test Result" class="Bool (엄격한)"("Colors [4]"=cluster{u32, u32}[] [{12369084, 12369084}, {12369084, 12369084}, {1985280, 1985280}, {1985280, 1985280}]) -> ()  [unwired: 2 in, 2 out]
        n17 = local write "Front Panel Data"(dbl[][] [] ("DevLoads")) -> ()
        n18 = Power Of 2(x=15.0) -> (2^x=w77:dbl)
        n19 = Multiply(x=w69, y=6) -> (x*y=w68:i32)
        n20 = Initialize Array(w77, 3, w68) -> (→"Base Accels":dbl[][])
        n21 = control-ref of="Prog Page #"() -> (w46:refnum<vi>)
        n22 = Initialize Array(3.0, 3, w68) -> (→"Six Plane Accels":dbl[][])
        n23 = global write "Gen2 FT Globals.vi" "Page Num"(w46) -> ()
        n24 = control-ref of="Transceiver Channel"() -> (w36:refnum<vi>)
        n25 = call "Read Config.vi"("error in (no error)"=w57, "Data In"=w58) -> ("error out"=w56:errorcluster, "Data Out"=w43:T8)  [unwired: 8 in]
        n26 = local write "Override 4th Test"(TRUE ("Overwrite 4th Test")) -> ()
        n27 = local write "Close Xsceiver"(w51) -> ()
        n28 = global write "Gen2 FT Globals.vi" "CustomCalFactors?"(w51) -> ()
        n29 = global write "Gen2 FT Globals.vi" "ZeroDev?"(w51) -> ()
        n30 = global write "Gen2 FT Globals.vi" "RawRxTx"(w51) -> ()
        n31 = local write "Estop"(w51) -> ()
        n32 = local write "ClearBuffer"(w51) -> ()
        n33 = local write "Test Device"(w51) -> ()
        n34 = global write "Gen2 FT Globals.vi" "Transceiver Ch"(w36) -> ()
        n35 = disable-structure shown="RUN_TIME_ENGINE==True" {
          disable-tunnel: [TRUE ("FTS Main?") FALSE ("FTS Main?")] -> w55
          frame condition #0 {
            # "Run Time\nUse Mark10"
          }
          frame condition #1 (active) {
            # "Development\ndon't use\nMark10"
          }
        }
        n36 = property on="CaptureButton" class="Bool (엄격한)"(error in=w56, "Visible"=FALSE, "DisabledEnum"=T21."Disabled" ("Disabled"), "Value"=FALSE ("CaptureButton")) -> (error out=w54:errorcluster)  [unwired: 1 in, 1 out]
        n37 = control-ref of="Operating Channel"() -> (w44:refnum<vi>)
        n38 = control-ref of="Target Channel"() -> (w40:refnum<vi>)
        n39 = Unbundle By Name(w43) -> ("Target Channel"=w39:string, "Operator Channel"=w42:string)
        n40 = property class="CmbBox (엄격한)"(reference=w40, "Value"=w39, "DisabledEnum"=T21."Disabled" ("Disabled")) -> ()  [unwired: 1 in, 2 out]
        n41 = property class="CmbBox"(reference=w44, "Value"=w42) -> ()  [unwired: 1 in, 2 out]
        n42 = Decimal String To Number(string=w39) -> (number=w38:i32)  [unwired: 2 in, 1 out]
        n43 = Get Date/Time In Seconds() -> (seconds since 1Jan1904=w53:timestamp)
        n44 = Decimal String To Number(string=w42) -> (number=w41:i32)  [unwired: 2 in, 1 out]
        n45 = Bundle By Name(cluster=w43, "Channels.Start Ch"=w48, "Channels.Operating Ch"=w41, "Channels.Transceiver Ch"=w48, "Target Information.Target Channel"=w38, "Use Mark10?"=w55, "Shutdown Counter"=w65, "DUT Parameters.Lot#"=w65, "Software Version"=w64, "Target Information.Target Serial#"=0 ("Target Serial#"), "NextState"=Gen2_FT_states."Timeout", "Scroll Message?"=TRUE, "MfgDate"=w53, "FTS Main?"=TRUE, "Program Retry"=FALSE) -> (w66:T8)
        "SoftwareVersion" <- w64
        "Device ON?" <- w51
        "Unit failed 3x Tests" <- w51
        "Accelerometer sample size" <- w69
        "Test Result" <- w51
        "Prog Page #" <- 0
      }
      frame "Read Support Data" {
        n46 = call "Load Support Script.vi"("error in (no error)"=w94, "Data In"=w93) -> ("error out"=w92:errorcluster, "Done?"=w90:bool, "Data Out"=w91:T8)  [unwired: 7 in]
        n47 = Select(t=Gen2_FT_states."Initialize Mark-10" ("Current State Out"), s=w90, f=Gen2_FT_states."Read Support Data" ("Current State Out")) -> (s? t:f=w88:T6)
      }
      frame "Initialize Mark-10" {
        # "Trys to connect with Mark-10 on the latest configuration port found in configuration \nfile: Mark-10ComPort.ini. If file does not exist the front panel control will be saved to\nthe folder"
        n48 = control-ref of="Mark-10 COM Port"() -> (w97:refnum<vi>)
        n49 = call <vilib>:"Clear Errors.vi"("error in (no error)"=w100) -> ("error out"=w96:errorcluster)  [unwired: 5 in, 1 out]
        n50 = call "Mark10 Inizialize.vi"("error in"=w96, "Data In"=w99, "Mark10"=w97) -> ("error out"=w101:errorcluster, "Data Out"=w98:T8, "Current State Out"=w95:T6)  [unwired: 6 in]
      }
      frame "Initialize Transceiver" {
        n51 = call "Initialize Transceiver.vi"("error in (no error)"=w109, "State-machine Local Variables"=w105) -> ("error out"=w108:errorcluster, "Rev String"=→"Rev String":string, "Initialized?"=w103:bool)  [unwired: 7 in]
        n52 = Select(t=Gen2_FT_states."Read Serial Lookup" ("Current State Out"), s=w103, f=Gen2_FT_states."Initialize Transceiver") -> (s? t:f=w102:T6)
      }
      frame "------UTILITIES------" {
        # "USED ONLY AS HEADER"
      }
      frame "Change DUT Channel" {
        n53 = call "DUT Change Channel.vi"("error in (no error)"=w116, "Data Cluster"=w114) -> ("error out"=w115:errorcluster, "Data Out"=w113:T8)  [unwired: 7 in, 1 out]
      }
      frame "Find RxTx Window" {
        n54 = control-ref of="This VI"() -> (w119:refnum<vi>)
        n55 = local read "Test Device"() -> (w124:bool)
        n56 = call "Find Window.vi"("error in (no error)"=w123, "This VI"=w119, "Testing?"=w124, "Main Data"=w126) -> ("error out"=w121:errorcluster, "Stop Testing?"=w122:bool, "Main Data"=w125:T8)  [unwired: 5 in]
        n57 = case shown="거짓" w122 {
          tunnel: w121 -> [w127 w130]
          tunnel: [w127 w129] -> w120
          frame False {
          }
          frame True {
            # "Testing Stopped"
            n58 = property on="Test Device" class="Bool (엄격한)"(error in=w130, "Val(Sgnl)"=FALSE ("Value (Signaling)")) -> (error out=w129:errorcluster)  [unwired: 1 in, 1 out]
          }
        }
      }
      frame "Reset Device" {
        n59 = call "Reset DUT.vi"("error in (no error)"=w133, "State-machine Local Variables in"=w135) -> ("error out"=w132:errorcluster, "State-machine Local Variables out"=w134:T8)  [unwired: 8 in]
      }
      frame "Scan Channels" {
        n60 = control-ref of="This VI"() -> (w136:refnum<vi>)
        n61 = call "Scan All Channels.vi"("error in (no error)"=w140, "VI in"=w136, "State-machine Local Variables in"=w137) -> ("error out"=w139:errorcluster, "State-machine Local Variables out"=w141:T8)  [unwired: 7 in]
      }
      frame "Read Serial Lookup" {
        n62 = Set Occurrence(w142) -> ()
        n63 = call "Read Serial Number Folder.vi"("error in"=w150, "Data IN"=w151) -> ("error out"=w146:errorcluster, "Current State Out"=w145:T6, "State-machine Local Variables out"=w149:T8)  [unwired: 7 in]
        n64 = Unbundle By Name(w149) -> ("Serial Table.Serial File Path"=→"Serial Folder Path":path, "Serial Table.[[Serial Lookup Table]]"=→"Serial Table Lookup":string[][])
        n65 = Bundle By Name(cluster=w149, "Message"="System Ready...") -> (w144:T8)
      }
      frame "Shutdown Device" {
        w154 = TRUE  # Clear?
        n66 = local write "Test Device"(FALSE ("Test Device")) -> ()
        n67 = local read "Device ON?"() -> (w157:bool)
        n68 = call "Shutdown DUT.vi"("error in (no error)"=w155, "Device On?"=w157, "Blast?"=FALSE, "Data In"=w160) -> ("error out"=w153:errorcluster, "State-machine Local Variables out"=w158:T8)  [unwired: 6 in]
        n69 = call "RxBuffer.vi"("Clear?"=w154, "error in (no error)"=w153) -> ("error out"=w152:errorcluster)  [unwired: 6 in, 11 out]
      }
      frame "ESTOP" {
        n70 = call "Mark10.vi"("Data In"=w163, "error in (no error)"=w168, "Action"=Mark10_states."Go Home") -> ("Done?"=w166:bool, "error out"=w167:errorcluster)  [unwired: 12 in, 3 out]
        n71 = Select(t=Gen2_FT_states."Timeout" ("Current State Out"), s=w166, f=Gen2_FT_states."ESTOP") -> (s? t:f=w162:T6)
      }
      frame "--------USER---------" {
        # "USED ONLY AS HEADER"
      }
      frame "Timeout", Default {
        n72 = event shown="[28] \"CaptureButton\": 값 변경" {
          selector: _ -> [_ _ _ _ _ _ _ _ _ _ _ _ _ _ _ _ _ _ _ _ _ _ _ _ _ _ _ _ _ _ _]
          dyn-events: _ -> [_ _ _ _ _ _ _ _ _ _ _ _ _ _ _ _ _ _ _ _ _ _ _ _ _ _ _ _ _ _ _]
          timeout: 5 -> [_ _ _ _ _ _ _ _ _ _ _ _ _ _ _ _ _ _ _ _ _ _ _ _ _ _ _ _ _ _ _]
          tunnel: [w211 Gen2_FT_states."Timeout" ("Current State Out") Gen2_FT_states."Timeout" ("Current State Out") Gen2_FT_states."Timeout" ("Current State Out") Gen2_FT_states."Timeout" ("Current State Out") Gen2_FT_states."Timeout" ("Current State Out") Gen2_FT_states."Timeout" ("Current State Out") Gen2_FT_states."Timeout" ("Current State Out") Gen2_FT_states."Timeout" ("Current State Out") Gen2_FT_states."Timeout" ("Current State Out") Gen2_FT_states."Exit" ("Current State Out") Gen2_FT_states."Read Serial Lookup" ("Current State Out") w364 w383 w389 Gen2_FT_states."MoveDown" ("Current State Out") Gen2_FT_states."MoveUp" ("Current State Out") w400 w405 Gen2_FT_states."Timeout" ("Current State Out") Gen2_FT_states."Timeout" ("Current State Out") Gen2_FT_states."Timeout" ("Current State Out") Gen2_FT_states."Timeout" ("Current State Out") w525 Gen2_FT_states."Timeout" ("Current State Out") Gen2_FT_states."Timeout" ("Current State Out") Gen2_FT_states."Timeout" ("Current State Out") Gen2_FT_states."Timeout" ("Current State Out") Gen2_FT_states."Timeout" ("Current State Out") Gen2_FT_states."Read Serial Lookup" ("Current State Out") Gen2_FT_states."Timeout" ("Current State Out")] -> w174
          tunnel: w180 -> [w210 w232 w238 w243 w249 w252 w268 w273 w280 w352 w355 w359 w363 w382 w388 w393 w396 w399 w404 w409 w440 w493 w518 w523 w578 w583 w589 w596 w615 w626 w631]
          tunnel: [w212 w230 w237 w241 w248 w251 w265 w270 w279 w351 w355 w359 w362 w382 w388 w393 w396 w399 w404 w412 w439 w493 w517 w522 w576 w581 w586 w590 w621 w624 w642] -> w177
          tunnel: w179 -> [w213 _ _ _ _ _ _ _ _ _ _ _ _ _ _ _ _ _ _ _ _ _ _ _ _ _ _ _ _ _ _]
          tunnel: w178 -> [_ _ _ _ _ _ _ _ _ _ _ _ _ _ _ _ _ _ _ _ _ _ _ w521 _ _ _ _ _ _ _]
          tunnel: w176 -> [w209 w231 w234 w242 w246 w254 w266 w271 w274 w350 w354 w358 w361 w381 w387 w392 w395 w398 w403 w410 w436 w492 w509 w520 w577 w582 w588 w594 w616 w625 w630]
          tunnel: [w209 w231 w234 w242 w246 w253 w266 w271 w274 w350 w354 w358 w360 w381 w387 w392 w395 w398 w403 w410 w435 w491 w509 w520 w577 w582 w588 w593 w616 w625 w629] -> w175
          event Timeout {
            n73 = event-data() -> ()  [unwired: 1 in, 2 out]
            n74 = Unbundle By Name(w210) -> ("G.Load"=→"Gauge Load":dbl, "G.Position"=→"Gauge Position":dbl, "NextState"=w204:T6, "Loading.[Forces]"=w184:dbl[], "[G.Loads]"=w185:dbl[], "[TotalLoads]"=w200:dbl[], "[CondyleLoads]"=w183:dbl[][], "[Errors]"=w186:dbl[][], "PCB Score"=→"PCB Score":i32, "AssyScore"=→"AssemScore":i32, "Channels.Transceiver Ch"=→"Transceiver Channel":u8, "Scroll Message?"=w182:bool)  [unwired: 1 out]
            n75 = Quotient & Remainder(x=w213, y=5) -> (x-y*floor(x/y)=w205:i32)  [unwired: 1 out]
            n76 = Transpose 2D Array(2D array=w186) -> (transposed array=w195:dbl[][])
            n77 = Build Array(w184, w185, w200) -> (w199:dbl[][])
            n78 = Transpose 2D Array(2D array=w183) -> (transposed array=w196:dbl[][])
            n79 = Equal To 0?(x=w205) -> (x = 0?=w189:bool)
            n80 = Build Array (concatenate)(w199, w196, w195) -> (w198:dbl[][])
            n81 = Transpose 2D Array(2D array=w198) -> (transposed array=→"Front Panel Data":dbl[][])
            n82 = call "MessageHandler.vi"("State-machine Local Variables"=w210) -> ("Message Out"=→"Message":string, "State-machine Local Variables out"=w190:T8)  [unwired: 7 in]
            n83 = And(x=w182, y=w189) -> (x .and. y?=w188:bool)
            n84 = case shown="참" w188 {
              frame False {
              }
              frame True {
                # "Scroll Message to Bottom"
                n85 = property on="Message" class="Str"("Text.Scroll Position"=inf) -> ()  [unwired: 2 in, 2 out]
              }
            }
            n86 = case shown="\"Timeout\"" w204 {
              selector: w204 -> [w221 w225]
              tunnel: [w221 w226] -> w211
              tunnel: w189 -> [_ w227]
              tunnel: w190 -> [w220 w224]
              tunnel: [w220 w224] -> w192
              frame Default {
              }
              frame "Timeout" {
                n87 = Wait Until Next ms Multiple(millisecond multiple=u32 50) -> ()  [unwired: 1 out]
                n88 = Select(t=Gen2_FT_states."Display Result" ("Current State Out"), s=w227, f=w225) -> (s? t:f=w226:T6)
              }
            }
            n89 = Unbundle By Name(w192) -> ("ScanTime"=w202:timestamp)
            n90 = Get Date/Time In Seconds() -> (seconds since 1Jan1904=w203:timestamp)
            n91 = Greater?(x=w203, y=w202) -> (0:w201:bool)
            n92 = case shown="참" w201 {
              tunnel: w192 -> [w215 w219]
              tunnel: [w215 w218] -> w212
              frame False {
              }
              frame True {
                n93 = Bundle By Name(cluster=w219, "Valid String?"=FALSE, "ScannedString"="") -> (w218:T8)
              }
            }
          }
          event "Clear Messages": Value Change {
            n94 = event-data() -> ()  [unwired: 1 in, 5 out]
            n95 = Bundle By Name(cluster=w232, "Clear Message"=TRUE) -> (w230:T8)
          }
          event Value Change {
            n96 = event-data() -> ()  [unwired: 1 in, 5 out]
            n97 = Decimal String To Number(string="Target Channel") -> (number=w235:i32)  [unwired: 2 in, 1 out]
            n98 = Bundle By Name(cluster=w238, "Target Information.Target Channel"=w235) -> (w237:T8)
          }
          event "Operator": Value Change {
            n99 = event-data() -> ()  [unwired: 1 in, 5 out]
            n100 = Bundle By Name(cluster=w243, "Operator"="Operator") -> (w241:T8)
          }
          event "Operating Channel": Value Change {
            n101 = event-data() -> ()  [unwired: 1 in, 5 out]
            n102 = Decimal String To Number(string="Operating Channel") -> (number=w244:i32)  [unwired: 2 in, 1 out]
            n103 = Bundle By Name(cluster=w249, "Channels.Operating Ch"=w244) -> (w248:T8)
          }
          event Value Change {
            w260 = TRUE ("RF Chip0 Enable")
            w259 = XceiverCmds."Set Channel" ("XceiverCmd")
            n104 = event-data() -> ()  [unwired: 1 in, 6 out]
            n105 = Decimal String To Number(string="Start Channel") -> (number=w250:i32)  [unwired: 2 in, 1 out]
            n106 = Concatenate Strings("RF Channel Changed to: ", "Start Channel") -> (w261:string)
            n107 = call "XceiverCmds.vi"("RF Chip0 Channel"=w250, "RF Chip1 Channel"=w250, "error in (no error)"=w254, "XceiverCmd"=w259) -> ("error out"=w258:errorcluster)  [unwired: 9 in, 2 out]
            n108 = Bundle By Name(cluster=w252, "Channels.Start Ch"=w250, "Channels.Transceiver Ch"=w250, "Message"=w261) -> (w251:T8)
            n109 = call "XceiverCmds.vi"("RF Chip0 Channel"=w250, "RF Chip0 Enable"=w260, "RF Chip1 Enable"=w260, "RF Chip1 Channel"=w250, "error in (no error)"=w258, "XceiverCmd"=w259) -> ("error out"=w257:errorcluster)  [unwired: 7 in, 2 out]
            n110 = call "RxBuffer.vi"("Clear?"=TRUE, "error in (no error)"=w257) -> ("error out"=w253:errorcluster)  [unwired: 6 in, 11 out]
          }
          event "Message": Mouse Enter {
            n111 = event-data() -> ()  [unwired: 1 in, 4 out]
            n112 = Bundle By Name(cluster=w268, "Scroll Message?"=FALSE ("Stop Scroll?")) -> (w265:T8)
          }
          event "Message": Mouse Leave {
            n113 = event-data() -> ()  [unwired: 1 in, 4 out]
            n114 = Bundle By Name(cluster=w273, "Scroll Message?"=TRUE ("Scroll?")) -> (w270:T8)
          }
          event Key Down {
            n115 = event-data() -> ("ScanCode"=w277:i16, "PlatMods"=w283:T25, "Char"=w278:i16)  [unwired: 1 in]
            n116 = Equal?(x=i16 37 ("ScanCode for \"k\""), y=w277) -> (x = y?=w284:bool)
            n117 = Unbundle By Name(w283) -> ("Ctrl"=w276:bool)
            n118 = And(x=w284, y=w276) -> (x .and. y?=w281:bool)
            n119 = case shown="거짓" w281 {
              tunnel: w280 -> [w287 w336]
              tunnel: [w286 w336] -> w279
              tunnel: w278 -> [w285 _]
              frame False {
                n120 = Unbundle By Name(w287) -> ("Valid String?"=w288:bool)
                n121 = case shown="거짓" w288 {
                  tunnel: w287 -> [w314 w334]
                  tunnel: [w289 w334] -> w286
                  tunnel: w285 -> [w297 _]
                  frame False {
                    n122 = Unbundle By Name(w314) -> ("ScanTime"=w304:timestamp, "ScannedString"=w313:string)
                    n123 = Get Date/Time In Seconds() -> (seconds since 1Jan1904=w296:timestamp)
                    n124 = case shown="\"\"" w313 {
                      selector: w313 -> [w325 w329]
                      tunnel: [w327 w332] -> w312
                      tunnel: w314 -> [w327 w333]
                      tunnel: w304 -> [w326 _]
                      tunnel: [w326 w330] -> w303
                      tunnel: [w325 w329] -> w302
                      tunnel: w296 -> [_ w328]
                      frame Default {
                      }
                      frame "" {
                        w331 = 5.0  # Allowed ScanTime (Sec)
                        # "Starting of string,\nso start timer"
                        n125 = Add(x=w328, y=w331) -> (x+y=w330:timestamp)
                        n126 = Bundle By Name(cluster=w333, "ScanTime"=w330) -> (w332:T8)
                      }
                    }
                    n127 = Type Cast(type="", x=w297) -> (*(type *) &x=w307:string)
                    n128 = Reverse String(1:w307) -> (0:w308:string)
                    n129 = String Subset(string=w308, length (rest)=1 ("length (rest)")) -> (substring=w301:string)  [unwired: 1 out]
                    n130 = case shown="기본" w301 {
                      selector: w301 -> [w316 _]
                      tunnel: [w316 _] -> w300
                      tunnel: [_ w317] -> w294
                      tunnel: w297 -> [_ w318]
                      frame ",", "-", ".", "/", "0", "1", "2", "3", "4", "5", "6", "7", "8", "9", ":", "A".."Z", "[", "]", "a".."z" {
                      }
                      frame Default {
                        n131 = Equal To 0?(x=w318) -> (x = 0?=w317:bool)
                      }
                    }
                    n132 = Greater?(x=w296, y=w303) -> (0:w295:bool)
                    n133 = Concatenate Strings(w302, w300) -> (w315:string)
                    n134 = call "BatchTest BoolValue Change.vi"("Value In"=w294) -> ("Value Changed?"=w292:bool, "Value Out"=w293:bool)  [unwired: 7 in, 2 out]
                    n135 = And(x=w293, y=w292) -> (x .and. y?=w291:bool)
                    n136 = Select(t="", s=w295, f=w315) -> (s? t:f=w299:string)
                    n137 = call "ValidateScan.vi"("LF?"=w291, "String In"=w299) -> ("Valid Format?"=w298:bool, "ScanData"=w305:T26, "String Out"=w306:string)  [unwired: 6 in, 1 out]
                    n138 = Bundle By Name(cluster=w312, "ScannedString"=w306, "Valid String?"=w298) -> (w290:T8)
                    n139 = case shown="참" w298 {
                      tunnel: w305 -> [_ w324]
                      tunnel: w290 -> [w319 w323]
                      tunnel: [w319 w322] -> w289
                      frame False {
                      }
                      frame True {
                        n140 = Unbundle By Name(w324) -> ("DeviceID"=w321:u32, "Mfg Date"=w320:timestamp)
                        n141 = Bundle By Name(cluster=w323, "LabelDevID"=w321, "MfgDate"=w320) -> (w322:T8)
                      }
                    }
                  }
                  frame True {
                  }
                }
              }
              frame True {
                # "1606, 808"
                # "1071, 808"
                # "1600, 710"
                n142 = control-ref of="This VI"() -> (w342:refnum<vi>)
                n143 = property class="VI"(reference=w342) -> (reference out=w344:refnum<vi>, "Front Panel.PanelBounds"=w343:T27)  [unwired: 1 in, 1 out]
                n144 = Unbundle By Name(w343) -> ("Right"=w341:i16, "Left"=w339:i16)
                n145 = Subtract(x=w341, y=w339) -> (x-y=w340:i16)
                n146 = case shown="기본" w340 {
                  tunnel: [i16 1071 i16 1606] -> w338
                  frame Default {
                  }
                  frame 1071 {
                  }
                }
                n147 = Add(x=w338, y=w339) -> (x+y=w337:i16)
                n148 = Bundle By Name(cluster=w343, "Right"=w337) -> (w335:T27)
                n149 = property class="VI"(reference=w344, "Front Panel.PanelBounds"=w335) -> ()  [unwired: 1 in, 2 out]
              }
            }
          }
          event "Shutdown Dev": Value Change {
            n150 = event-data() -> ()  [unwired: 1 in, 5 out]
            n151 = Bundle By Name(cluster=w352, "Message"="Attempting to turn OFF the Device, please wait...", "Shutdown Counter"=u32 0, "NextState"=Gen2_FT_states."Shutdown Device") -> (w351:T8)
          }
          event "Exit": Value Change {
            n152 = event-data() -> ()  [unwired: 1 in, 5 out]
          }
          event "Refresh Button": Value Change {
            n153 = event-data() -> ()  [unwired: 1 in, 6 out]
          }
          event Value Change {
            n154 = event-data() -> ("NewVal"=w365:T5)  [unwired: 1 in, 4 out]
            n155 = case shown="참" w365 {
              tunnel: [Gen2_FT_states."End Test" ("Current State Out") Gen2_FT_states."ESTOP" ("Current State Out")] -> w364
              tunnel: w363 -> [w367 w371]
              tunnel: [w367 w379] -> w362
              tunnel: w361 -> [w366 w373]
              tunnel: [w366 w372] -> w360
              frame False {
                n156 = property on="Message" class="Str"("Blinking"=FALSE) -> ()  [unwired: 2 in, 2 out]
              }
              frame True {
                w375 = T21."Disabled" ("Disabled")
                w370 = T21."Disabled and Grayed Out" ("Disabled")
                w376 = "EMERGENCY STOP BUTTON IS ENABLED..." ("Message")
                n157 = property on="Target Serial#:" class="DigNum (엄격한)"("DisabledEnum"=w375) -> ()  [unwired: 2 in, 2 out]
                n158 = property on="Shutdown Dev" class="Bool"("DisabledEnum"=w375) -> ()  [unwired: 2 in, 2 out]
                n159 = property on="Scan Channels" class="Bool"("DisabledEnum"=w370) -> ()  [unwired: 2 in, 2 out]
                n160 = property on="Start Channel" class="CmbBox (엄격한)"("DisabledEnum"=w370) -> ()  [unwired: 2 in, 2 out]
                n161 = property on="Operating Channel" class="CmbBox"("DisabledEnum"=w370) -> ()  [unwired: 2 in, 2 out]
                n162 = call "Mark10.vi"("Data In"=w371, "error in (no error)"=w373, "Action"=Mark10_states."Stop Motor") -> ("error out"=w372:errorcluster)  [unwired: 12 in, 4 out]
                n163 = property on="Message" class="Str"("Blinking"=TRUE, "Value"=w376) -> ()  [unwired: 2 in, 2 out]
                n164 = Bundle By Name(cluster=w371, "Message"=w376, "Test Result"=FALSE) -> (w379:T8)
              }
            }
          }
          event "StopMotor": Value Change {
            n165 = event-data() -> ("NewVal"=w384:bool)  [unwired: 1 in, 4 out]
            n166 = case shown="거짓" w384 {
              tunnel: [Gen2_FT_states."Timeout" ("Current State Out") Gen2_FT_states."Stop Motor" ("Current State Out")] -> w383
              frame False {
              }
              frame True {
              }
            }
          }
          event "Home": Value Change {
            n167 = event-data() -> ("NewVal"=w390:bool)  [unwired: 1 in, 4 out]
            n168 = case shown="참" w390 {
              tunnel: [_ Gen2_FT_states."Go Home" ("Current State Out")] -> w389
              frame False {
              }
              frame True {
              }
            }
          }
          event "MoveDown": Value Change {
            n169 = event-data() -> ()  [unwired: 1 in, 5 out]
          }
          event "MoveUp": Value Change {
            n170 = event-data() -> ()  [unwired: 1 in, 5 out]
          }
          event "GotoLoad": Value Change {
            n171 = event-data() -> ("NewVal"=w401:bool)  [unwired: 1 in, 4 out]
            n172 = case shown="참" w401 {
              tunnel: [_ Gen2_FT_states."Goto Load" ("Current State Out")] -> w400
              frame False {
              }
              frame True {
              }
            }
          }
          event "GotoPosition": Value Change {
            n173 = event-data() -> ("NewVal"=w406:bool)  [unwired: 1 in, 4 out]
            n174 = case shown="참" w406 {
              tunnel: [_ Gen2_FT_states."Goto Position" ("Current State Out")] -> w405
              frame False {
              }
              frame True {
              }
            }
          }
          event "Override 4th Test": Value Change {
            n175 = event-data() -> ()  [unwired: 1 in, 6 out]
            n176 = Unbundle By Name(w409) -> ("Target Information.Target Serial#"=w408:i32)
            n177 = Equal To 0?(x=w408) -> (x = 0?=w413:bool)
            n178 = case shown="거짓" w413 {
              tunnel: w409 -> [w418 w434]
              tunnel: [w419 w433] -> w412
              tunnel: w408 -> [w427 _]
              frame False {
                n179 = call <vilib>:"Application Directory.vi"() -> ("Application Directory"=w430:path)
                n180 = Build Path(base path=w430, name or relative path=path "SerialFails.ini") -> (appended path=w428:path)
                n181 = call <vilib>:"Open Config Data.vi"("configuration file path"=w428) -> ("error out"=w423:errorcluster, "refnum"=w426:T28)  [unwired: 8 in, 1 out]
                n182 = Number To Decimal String(number=w427) -> (decimal integer string=w416:string)  [unwired: 1 in]
                n183 = call-poly <vilib>:"Write Key.vi"("section"=w416, "error in (no error)"=w423, "value"=0, "key"="RunCount", "refnum"=w426) -> ("error out"=w420:errorcluster, "refnum out"=w421:T28)  [unwired: 4 in, 1 out]
                n184 = Concatenate Strings("Serial Number: " ("Message"), w416, " has been overridden" ("string")) -> (w415:string)
                n185 = local write "Override 4th Test"(TRUE ("Overwrite 4th Test")) -> ()
                n186 = Bundle By Name(cluster=w418, "Message"=w415) -> (w419:T8)
                n187 = call <vilib>:"Close Config Data.vi"("error in (no error)"=w420, "refnum"=w421) -> ()  [unwired: 8 in, 2 out]
              }
              frame True {
                n188 = Bundle By Name(cluster=w434, "Message"="Enter a Serial Number to Clear") -> (w433:T8)
                n189 = local write "Override 4th Test"(TRUE ("Overwrite 4th Test")) -> ()
              }
            }
          }
          event "Device ON?": Value Change {
            n190 = event-data() -> ("NewVal"=w438:bool)  [unwired: 1 in]
            n191 = case shown="참" w438 {
              tunnel: w440 -> [w446 w449]
              tunnel: [w445 w450] -> w439
              tunnel: w436 -> [w443 w447]
              tunnel: [w442 w447] -> w435
              frame False {
                w441 = TRUE  # Clear?
                n192 = Bundle By Name(cluster=w446, "RXTX Window Found?"=FALSE) -> (w445:T8)
                n193 = call "RxBuffer.vi"("Clear?"=w441, "error in (no error)"=w443) -> ("error out"=w442:errorcluster)  [unwired: 6 in, 11 out]
              }
              frame True {
                n194 = call "RxBuffer.vi"() -> ("DeviceParameters"=w451:T29, "New Data"=w448:bool)  [unwired: 8 in, 10 out]
                n195 = case shown="참" w448 {
                  selector: w448 -> [_ w459]
                  tunnel: w451 -> [_ w456]
                  tunnel: [w454 w458] -> w450
                  tunnel: w449 -> [w454 w457]
                  frame False {
                    n196 = property on="Device ON?" class="Bool (엄격한)"("BoolText.Text"="OFF" ("Boolean Text.Text")) -> ()  [unwired: 2 in, 2 out]
                    n197 = local write "Device ON?"(FALSE ("Device ON?")) -> ()
                  }
                  frame True {
                    n198 = Unbundle By Name(w456) -> ("GotCal"=w455:bool)
                    n199 = global write "Gen2 FT Globals.vi" "ZeroDev?"(w459) -> ()
                    n200 = property on="Device ON?" class="Bool (엄격한)"("BoolText.Text"="ON" ("Boolean Text.Text")) -> ()  [unwired: 2 in, 2 out]
                    n201 = case shown="참" w455 {
                      tunnel: [w465 w473] -> w458
                      tunnel: w457 -> [w466 w471]
                      tunnel: w456 -> [_ w467]
                      frame False {
                        w463 = "DUT Calibration was not received... " ("message")
                        n202 = One Button Dialog(message=w463) -> ()  [unwired: 1 in, 1 out]
                        n203 = Concatenate Strings(w463, "  Attempting to Shutdown DUT" ("string")) -> (w462:string)
                        n204 = Bundle By Name(cluster=w466, "Message"=w462, "NextState"=Gen2_FT_states."Shutdown Device") -> (w465:T8)
                      }
                      frame True {
                        n205 = call "Device On.vi"("DeviceParameters"=w467, "Data In"=w471) -> ("Data Out"=w470:T8)  [unwired: 9 in]
                        n206 = Unbundle By Name(w470) -> ("RXTX Window Found?"=w472:bool, "DUT Parameters.DeviceID"=w469:u32)
                        n207 = call "Device Family Change.vi"("Device ID"=w469) -> ("New Family"=w468:bool)  [unwired: 10 in]
                        n208 = case shown="거짓" w472 {
                          tunnel: [w477 w480] -> w473
                          tunnel: w470 -> [w476 w480]
                          frame False {
                            n209 = Bundle By Name(cluster=w476, "Message"="Attempting to Find RxTx Window. Please wait this could take up to 30 seconds", "NextState"=Gen2_FT_states."Find RxTx Window") -> (w477:T8)
                          }
                          frame True {
                          }
                        }
                        n210 = case shown="참" w468 {
                          frame False {
                          }
                          frame True {
                            n211 = property on="Correction Factor" class="Str"("Val(Sgnl)"="" ("Value (Signaling)")) -> ()  [unwired: 2 in, 2 out]
                            n212 = One Button Dialog(message="New family of Device Types detected.\nPlease enter a new Correction Factor") -> ()  [unwired: 1 in, 1 out]
                          }
                        }
                      }
                    }
                  }
                }
              }
            }
          }
          event "Blast Shutdown": Value Change {
            n213 = event-data() -> ()  [unwired: 1 in, 6 out]
            n214 = local read "Streaming Serial Number"() -> (w484:u32)
            n215 = Number To Decimal String(number=w484) -> (decimal integer string=w482:string)  [unwired: 1 in]
            n216 = Concatenate Strings("Do you want to shutdown this DUT: " ("message"), w482) -> (w481:string)
            n217 = Two Button Dialog(message=w481, 1:"Custom" ("F button name (\"Cancel\")"), 2:"Yes" ("T button name (\"OK\")")) -> (T button?=w485:bool)
            n218 = case shown="참" w485 {
              tunnel: [w495 TRUE ("Shutdown")] -> w490
              tunnel: [w494 w497] -> w489
              tunnel: w484 -> [_ w497]
              frame False {
                n219 = call "Enter Serial Number"() -> ("Serial Number"=w494:dbl, "Shutdown"=w495:bool)  [unwired: 17 in, 1 out]
              }
              frame True {
              }
            }
            n220 = case shown="참" w490 {
              tunnel: w492 -> [w498 w502]
              tunnel: [w498 w501] -> w491
              tunnel: w489 -> [_ w500]
              frame False {
              }
              frame True {
                n221 = for {
                  N: 6 -> [_]
                  tunnel: w500 -> [w504]
                  shift-right: [w505] -> w501
                  shift-left: w502 -> [w506]
                  n222 = call "Shutdown Device.vi"("error in (no error)"=w506, "Blast? (F)"=TRUE, "Serial Number"=w504) -> ("error out"=w505:errorcluster)  [unwired: 7 in, 1 out]
                  n223 = Wait (ms)(milliseconds to wait=u32 200) -> ()  [unwired: 1 out]
                }
              }
            }
          }
          event "Reset Device": Value Change {
            n224 = event-data() -> ()  [unwired: 1 in, 6 out]
            n225 = local read "Device ON?"() -> (w508:bool)
            n226 = Select(t="Attempting to reset device", s=w508, f="No Device Detected") -> (s? t:f=w516:string)
            n227 = Select(t=Gen2_FT_states."Reset Device" ("NextState"), s=w508, f=Gen2_FT_states."Timeout") -> (s? t:f=w510:T6)
            n228 = Bundle By Name(cluster=w518, "Message"=w516, "NextState"=w510) -> (w517:T8)
          }
          event "Test Device": Value Change {
            n229 = event-data() -> ("NewVal"=w524:bool)  [unwired: 1 in]
            n230 = property on="Test Result" class="Bool (엄격한)"("Colors [4]"=cluster{u32, u32}[] [{12369084, 12369084}, {12369084, 12369084}, {1985280, 1985280}, {1985280, 1985280}]) -> ()  [unwired: 2 in, 2 out]
            n231 = case shown="참" w524 {
              tunnel: [w534 w547] -> w525
              tunnel: w523 -> [w526 w545]
              tunnel: [w536 w546] -> w522
              tunnel: w521 -> [_ w543]
              frame False {
                w534 = Gen2_FT_states."Timeout" ("Current State Out")
                n232 = call "Mark10.vi"("Data In"=w526, "Action"=Mark10_states."Stop Motor") -> ("error out"=w528:errorcluster)  [unwired: 13 in, 4 out]
                n233 = call "Mark10.vi"("Data In"=w526, "error in (no error)"=w528, "Action"=Mark10_states."Go Home") -> ()  [unwired: 12 in, 5 out]
                n234 = global write "Gen2 FT Globals.vi" "RawRxTx"(FALSE ("RawRxTx")) -> ()
                n235 = Bundle By Name(cluster=w526, "Message"="Device programming cancelled...", "NextState"=w534, "Test Result"=FALSE ("Result"), "Result String"="Programming Cancelled", "NextState"=Gen2_FT_states."End Test" ("Current State Out")) -> (w536:T8)
              }
              frame True {
                n236 = Unbundle By Name(w545) -> ("Correction Factor"=w539:string, "Serial Table.Valid Serial?"=w544:bool)
                n237 = local read "Device ON?"() -> (w540:bool)
                n238 = Not(x=w543) -> (.not. x?=w541:T5)
                n239 = Empty String/Path?(string/path=w539) -> (empty?=w537:bool)
                n240 = Not(x=w537) -> (.not. x?=w538:bool)
                n241 = Compound Arithmetic op=AND(w538, w544, w541, w540) -> (w542:T5)
                n242 = case shown="참" w542 {
                  tunnel: [Gen2_FT_states."Timeout" ("Current State Out") w565] -> w547
                  tunnel: w545 -> [w563 w571]
                  tunnel: [w560 w570] -> w546
                  tunnel: w543 -> [w562 _]
                  tunnel: w540 -> [w554 _]
                  tunnel: w537 -> [w552 _]
                  frame False {
                    w548 = T21."Enabled" ("Disabled")
                    n243 = Not(x=w554) -> (.not. x?=w553:bool)
                    n244 = local write "Test Device"(FALSE ("StartTest")) -> ()
                    n245 = Select(t="Please release E-Stop...", s=w562, f="The Serial Number is not valid") -> (s? t:f=w558:string)
                    n246 = Select(t="Please Turn On a Device", s=w553, f=w558) -> (s? t:f=w551:string)
                    n247 = Select(t="Please Enter a Correction Factor", s=w552, f=w551) -> (s? t:f=w549:string)
                    n248 = property on="Start Channel" class="CmbBox (엄격한)"("DisabledEnum"=w548) -> ()  [unwired: 2 in, 2 out]
                    n249 = property on="Operating Channel" class="CmbBox"("DisabledEnum"=w548) -> ()  [unwired: 2 in, 2 out]
                    n250 = property on="Target Serial#:" class="DigNum (엄격한)"("DisabledEnum"=w548) -> ()  [unwired: 2 in, 2 out]
                    n251 = property on="Shutdown Dev" class="Bool"("DisabledEnum"=w548) -> ()  [unwired: 2 in, 2 out]
                    n252 = property on="Scan Channels" class="Bool"("DisabledEnum"=w548) -> ()  [unwired: 2 in, 2 out]
                    n253 = property on="Correction Factor" class="Str"("DisabledEnum"=w548) -> ()  [unwired: 2 in, 2 out]
                    n254 = Bundle By Name(cluster=w563, "Message"=w549) -> (w560:T8)
                  }
                  frame True {
                    w573 = T21."Disabled" ("Disabled")
                    w572 = T21."Disabled and Grayed Out" ("Disabled")
                    # "Inject Support scrip. If start ch is equal to operating ch\njump right into testing. If not Change DUT Channel"
                    # "Device will always be transmitting. Go to testing State"
                    n255 = call "Save General Data.vi"("Data Cluster"=w571) -> ("Data Out"=w570:T8)  [unwired: 7 in, 1 out]
                    n256 = Unbundle By Name(w570) -> ("Channels.Start Ch"=w569:u8, "Channels.Operating Ch"=w568:u8)
                    n257 = property on="Shutdown Dev" class="Bool"("DisabledEnum"=w573) -> ()  [unwired: 2 in, 2 out]
                    n258 = property on="Target Serial#:" class="DigNum (엄격한)"("DisabledEnum"=w573) -> ()  [unwired: 2 in, 2 out]
                    n259 = property on="Correction Factor" class="Str"("DisabledEnum"=w572) -> ()  [unwired: 2 in, 2 out]
                    n260 = Equal?(x=w569, y=w568) -> (x = y?=w564:bool)
                    n261 = property on="Operating Channel" class="CmbBox"("DisabledEnum"=w572) -> ()  [unwired: 2 in, 2 out]
                    n262 = property on="Scan Channels" class="Bool"("DisabledEnum"=w572) -> ()  [unwired: 2 in, 2 out]
                    n263 = property on="Start Channel" class="CmbBox (엄격한)"("DisabledEnum"=w572) -> ()  [unwired: 2 in, 2 out]
                    n264 = Select(t=Gen2_FT_states."Start Test" ("Current State Out"), s=w564, f=Gen2_FT_states."Change DUT Channel" ("Current State Out")) -> (s? t:f=w565:T6)
                  }
                }
              }
            }
          }
          event "Eng Log?": Value Change {
            n265 = event-data() -> ()  [unwired: 1 in, 6 out]
            n266 = Bundle By Name(cluster=w578, "Engr Log?"="Eng Log?") -> (w576:T8)
          }
          event "Correction Factor": Value Change {
            n267 = event-data() -> ()  [unwired: 1 in, 6 out]
            n268 = Bundle By Name(cluster=w583, "Correction Factor"="Correction Factor") -> (w581:T8)
          }
          event "Scan Channels": Value Change {
            n269 = event-data() -> ()  [unwired: 1 in, 6 out]
            n270 = Bundle By Name(cluster=w589, "Message"="Scanning for Devices. Please Wait. ", "NextState"=Gen2_FT_states."Scan Channels" ("Current State Out")) -> (w586:T8)
          }
          event "Target Serial#:": Value Change {
            n271 = event-data() -> ()  [unwired: 1 in, 6 out]
            n272 = call "Serial Table Lookup.vi"("error in (no error)"=w594, "Target Serial#:"="Target Serial#:", "Data IN"=w596) -> ("error out"=w593:errorcluster, "Valid Serial"=w592:bool, "State-machine Local Variables out"=w591:T8)  [unwired: 6 in]
            n273 = case shown="참" w592 {
              tunnel: w591 -> [w598 w607]
              tunnel: [w598 w608] -> w590
              frame False {
                # "Issues with serial number file. Operator was warned of issue with\npop up message. \n\nNo device information to update or image to display"
              }
              frame True {
                # "By Index:\n0 - Serial Number\n1 - Lot Number\n2 - Brand\n3 - Type\n4 - Device ID"
                n274 = Unbundle By Name(w607) -> ("Serial Table.Serial Device Info"=w609:string[])
                n275 = Index Array(array=w609) -> (element #1=w606:string, element #2=w604:string, element #3=w602:string, element #4=w601:string, element #5=w600:string)  [unwired: 5 in]
                "Brand:" <- w602
                "DeviceType:" <- w601
                "Lot#:" <- w604
                "DeviceID:" <- w600
                n276 = Decimal String To Number(string=w606) -> (number=w605:i32)  [unwired: 2 in, 1 out]
                n277 = Decimal String To Number(string=w604) -> (number=w603:i32)  [unwired: 2 in, 1 out]
                n278 = Decimal String To Number(string=w600) -> (number=w599:i32)  [unwired: 2 in, 1 out]
                n279 = call "LoadDeviceImage.vi"("DevID"=w599) -> ("AppBGpic"=→"Device Image":picture, "Image Found?"=w610:bool)  [unwired: 9 in]
                n280 = Bundle By Name(cluster=w607, "Target Information.Target Serial#"=w605, "Target Information.Target Lot#"=w603, "Target Information.Target Brand"=w602, "Target Information.Target DeviceType"=w601, "Target Information.Target DevID"=w599) -> (w608:T8)
                n281 = property on="Device Image" class="Pict"("Visible"=w610) -> ()  [unwired: 2 in, 2 out]
              }
            }
          }
          event "CaptureButton": Value Change {
            n282 = event-data() -> ()  [unwired: 1 in, 6 out]
            n283 = property on="CaptureButton" class="Bool (엄격한)"("Visible"=FALSE, "DisabledEnum"=T21."Disabled" ("Disabled"), "Value"=FALSE ("CaptureButton")) -> ()  [unwired: 2 in, 2 out]
            n284 = Unbundle By Name(w615) -> ("Angle Test Step"=w614:T30)
            n285 = Increment(x=w614) -> (x+1=w613:T30)
            n286 = Bundle By Name(cluster=w615, "Angle Test Step"=w613, "NextState"=Gen2_FT_states."Angle Test") -> (w621:T8)
          }
          event "Change Path": Value Change {
            n287 = event-data() -> ()  [unwired: 1 in, 6 out]
            n288 = Bundle By Name(cluster=w626, "Serial Table.Serial File Path"=path "") -> (w624:T8)
          }
          event "Mark-10 COM Port": Value Change {
            n289 = event-data() -> ()  [unwired: 1 in, 2 out]
            n290 = call <vilib>:"Application Directory.vi"() -> ("Application Directory"=w640:path)
            n291 = Build Path(base path=w640, name or relative path=path "Mark-10ComPort.ini") -> (appended path=w638:path)
            n292 = Bundle By Name(cluster=w631, "COM Port"="Mark-10 COM Port") -> (w628:T8)
            n293 = call <vilib>:"Open Config Data.vi"("configuration file path"=w638) -> ("refnum"=w637:T28)  [unwired: 8 in, 2 out]
            n294 = call-poly <vilib>:"Write Key.vi"("section"="Mark-10 Com Port", "error in (no error)"=w630, "value"="Mark-10 COM Port", "key"="Com", "refnum"=w637) -> ("error out"=w633:errorcluster, "refnum out"=w634:T28)  [unwired: 4 in, 1 out]
            n295 = call <vilib>:"Close Config Data.vi"("error in (no error)"=w633, "refnum"=w634) -> ("error out"=w629:errorcluster)  [unwired: 8 in, 1 out]
            n296 = call "Mark10.vi"("Data In"=w628, "Action"=Mark10_states."Initialize") -> ()  [unwired: 13 in, 5 out]
            n297 = Bundle By Name(cluster=w628, "Message"="System Ready... Please Turn on device before starting test") -> (w642:T8)
          }
        }
        n298 = Get Date/Time In Seconds() -> (seconds since 1Jan1904=→"Time:":timestamp)
      }
      frame "-----PROGRAM-----" {
        # "USED ONLY AS HEADER"
      }
      frame "Program Device" {
        # ">> Batt Check"
        n299 = call "Program Device Main.vi"("error in (no error)"=w651, "Data In"=w650) -> ("error out"=w648:errorcluster, "Data Out"=w647:T8)  [unwired: 8 in]
      }
      frame "------MARK10--------" {
        # "USED ONLY AS HEADER"
      }
      frame "Go Home" {
        n300 = call "Mark10.vi"("Data In"=w659, "error in (no error)"=w669, "Action"=Mark10_states."Go Home") -> ("Live Load"=w665:dbl, "Live Position"=w666:dbl, "Done?"=w662:bool, "error out"=w668:errorcluster)  [unwired: 12 in, 1 out]
        n301 = Bundle By Name(cluster=w659, "Homed?"=TRUE, "G.Load"=w665, "G.Position"=w666, "Test Result"=FALSE) -> (w663:T8)
        n302 = Select(t=Gen2_FT_states."Timeout" ("Current State Out"), s=w662, f=Gen2_FT_states."Go Home" ("NextState")) -> (s? t:f=w655:T6)
        n303 = Bundle By Name(cluster=w663, "NextState"=Gen2_FT_states."Timeout" ("Current State Out")) -> (w667:T8)
      }
      frame "MoveUp" {
        n304 = Compound Arithmetic op=AND("MoveUp", invert w676) -> (w677:T5)
        n305 = case shown="참" w677 {
          tunnel: w683 -> [w687 w695]
          tunnel: [w686 w694] -> w682
          tunnel: [w685 w689] -> w672
          tunnel: [w684 w693] -> w674
          tunnel: w673 -> [w684 w690]
          frame False {
            n306 = call "Mark10.vi"("Data In"=w684, "error in (no error)"=w687, "Action"=Mark10_states."Stop Motor") -> ("Done?"=w685:bool, "error out"=w686:errorcluster)  [unwired: 12 in, 3 out]
          }
          frame True {
            n307 = call "Mark10.vi"("Data In"=w690, "error in (no error)"=w695, "Action"=Mark10_states."Move Up") -> ("Live Load"=w691:dbl, "Live Position"=w692:dbl, "Done?"=w689:bool, "error out"=w694:errorcluster)  [unwired: 12 in, 1 out]
            n308 = Bundle By Name(cluster=w690, "G.Load"=w691, "G.Position"=w692) -> (w693:T8)
          }
        }
        n309 = Compound Arithmetic op=OR(invert "MoveUp", w672) -> (w678:bool)
        n310 = Bundle By Name(cluster=w674, "NextState"=Gen2_FT_states."Timeout") -> (w681:T8)
        n311 = Select(t=Gen2_FT_states."Timeout" ("Current State Out"), s=w678, f=Gen2_FT_states."MoveUp" ("NextState")) -> (s? t:f=w670:T6)
      }
      frame "MoveDown" {
        n312 = Compound Arithmetic op=AND("MoveDown", invert w703) -> (w704:T5)
        n313 = case shown="참" w704 {
          tunnel: w710 -> [w714 w722]
          tunnel: [w713 w721] -> w709
          tunnel: [w712 w720] -> w699
          tunnel: [w711 w719] -> w702
          tunnel: w701 -> [w711 w716]
          frame False {
            n314 = call "Mark10.vi"("Data In"=w711, "error in (no error)"=w714, "Action"=Mark10_states."Stop Motor") -> ("Done?"=w712:bool, "error out"=w713:errorcluster)  [unwired: 12 in, 3 out]
          }
          frame True {
            n315 = call "Mark10.vi"("Data In"=w716, "error in (no error)"=w722, "Action"=Mark10_states."Move Down") -> ("Live Load"=w717:dbl, "Live Position"=w718:dbl, "Done?"=w720:bool, "error out"=w721:errorcluster)  [unwired: 12 in, 1 out]
            n316 = Bundle By Name(cluster=w716, "G.Load"=w717, "G.Position"=w718) -> (w719:T8)
          }
        }
        n317 = Compound Arithmetic op=OR(invert "MoveDown", w699) -> (w705:bool)
        n318 = Select(t=Gen2_FT_states."Timeout" ("Current State Out"), s=w705, f=Gen2_FT_states."MoveDown" ("NextState")) -> (s? t:f=w697:T6)
        n319 = Bundle By Name(cluster=w702, "NextState"=Gen2_FT_states."Timeout") -> (w708:T8)
      }
      frame "Goto Load" {
        n320 = case shown="참" w726 {
          tunnel: w734 -> [w742 w747]
          tunnel: [w741 w746] -> w733
          tunnel: [w740 w745] -> w727
          tunnel: [w738 w744] -> w729
          tunnel: w728 -> [w735 w744]
          frame False {
            n321 = call "Mark10.vi"("Requested Load"="Load(lbs):", "Data In"=w735, "error in (no error)"=w742, "Action"=Mark10_states."Stop @ Load") -> ("Live Load"=w737:dbl, "Live Position"=w736:dbl, "Done?"=w740:bool, "error out"=w741:errorcluster)  [unwired: 11 in, 1 out]
            n322 = Bundle By Name(cluster=w735, "G.Load"=w737, "G.Position"=w736) -> (w738:T8)
          }
          frame True {
            n323 = call "Mark10.vi"("Data In"=w744, "error in (no error)"=w747, "Action"=Mark10_states."Stop Motor") -> ("Done?"=w745:bool, "error out"=w746:errorcluster)  [unwired: 12 in, 3 out]
          }
        }
        n324 = Select(t=Gen2_FT_states."Timeout" ("Current State Out"), s=w727, f=Gen2_FT_states."Goto Load" ("NextState")) -> (s? t:f=w730:T6)
        n325 = Bundle By Name(cluster=w729, "NextState"=w730) -> (w732:T8)
      }
      frame "Goto Position" {
        n326 = case shown="거짓" w750 {
          tunnel: w759 -> [w768 w773]
          tunnel: [w767 w772] -> w758
          tunnel: [w766 w771] -> w751
          tunnel: [w765 w770] -> w753
          tunnel: w752 -> [w761 w770]
          frame False {
            n327 = call "Mark10.vi"("Data In"=w761, "Requested Position"="Position(inch)", "Accuracy \nTest?"=FALSE, "error in (no error)"=w768, "Action"=Mark10_states."Goto Position") -> ("Live Load"=w764:dbl, "Live Position"=w763:dbl, "Done?"=w766:bool, "error out"=w767:errorcluster)  [unwired: 10 in, 1 out]
            n328 = Bundle By Name(cluster=w761, "G.Load"=w764, "G.Position"=w763) -> (w765:T8)
          }
          frame True {
            n329 = call "Mark10.vi"("Data In"=w770, "error in (no error)"=w773, "Action"=Mark10_states."Stop Motor") -> ("Done?"=w771:bool, "error out"=w772:errorcluster)  [unwired: 12 in, 3 out]
          }
        }
        n330 = Select(t=Gen2_FT_states."Timeout" ("Current State Out"), s=w751, f=Gen2_FT_states."Goto Position" ("NextState")) -> (s? t:f=w755:T6)
        n331 = Bundle By Name(cluster=w753, "NextState"=w755) -> (w757:T8)
      }
      frame "Stop Motor" {
        w779 = FALSE ("Blinking")
        w775 = Gen2_FT_states."Timeout" ("Current State Out")
        n332 = property on="Message" class="Str"("Blinking"=w779) -> ()  [unwired: 2 in, 2 out]
        n333 = global write "Gen2 FT Globals.vi" "ZeroDev?"(w779) -> ()
        n334 = call "Mark10.vi"("Data In"=w777, "error in (no error)"=w783, "Action"=Mark10_states."Stop Motor") -> ("Live Load"=w780:dbl, "Live Position"=w781:dbl, "error out"=w782:errorcluster)  [unwired: 12 in, 2 out]
        n335 = Bundle By Name(cluster=w777, "NextState"=w775, "G.Load"=w780, "G.Position"=w781) -> (w776:T8)
      }
      frame "---------TESTS--------" {
        # "USED ONLY AS HEADER"
      }
      frame "Start Test" {
        w787 = 0
        # "Initialize the test here. Jump to First Test"
        # "True unless proven otherwise"
        # "Initialize all Tests"
        # "True unless proven otherwise"
        n336 = Bundle By Name(cluster=w793, "Angle Test Step"=enum16{"Initialize", "Get X", "Get Y", "Get Z"}."Initialize", "Batt Test Step"=Batt_Cap_Steps."Initialize" ("Batt Capture State"), "Loading.Loading Step"=Load_Step."Initialize Test" ("Load Step"), "Test Result"=TRUE, "Programming Step"=Iniial_Device_Programming."Load EEPROM", "Final Program?"=TRUE, "Result String"="Test Passed" ("Error Message"), "Pass/Fail #"="", "Programming Mode"=ProgramStageControl."Scales" ("Programming Step"), "Program Retry"=FALSE, "New Data Program"=TRUE, "Page#"=w787, "NFHU Pass?"=TRUE, "Cal Cycle#"=w787, "Cal Retry?"=FALSE, "LA Cycle#"=w787, "Shim#"=w787) -> (w795:T8)
        n337 = local write "Prog Page #"(w787) -> ()
      }
      frame "Angle Test" {
        # ">>Move to Load Test"
        n338 = control-ref of="CaptureButton"() -> (w806:refnum<vi>)
        n339 = call "Accel Capture.vi"("Capture Button Ref"=w806, "Data IN"=w808) -> ("Data Out"=w807:T8)  [unwired: 9 in]
      }
      frame "Load Test" {
        # ">>Move to Load Accuracy"
        n340 = control-ref of="Test Result"() -> (w810:refnum<vi>)
        n341 = call "Load Test.vi"("error in (no error)"=w817, "Test Result 2"=w810, "Data In"=w813) -> ("error out"=w815:errorcluster, "LoadSensors"=→"Adj.Data":dbl[], "State-machine Local Variables out"=w816:T8, "Raw Data"=w812:u16[])  [unwired: 5 in]
        n342 = local write "RawData"(w812) -> ()
      }
      frame "Load Accuracy Test" {
        # ">>>Move to Program DUT"
        # "Insert Load Accuracy Test subvi here"
        n343 = call "Load Accuracy Test.vi"("error in"=w824, "Data In"=w823) -> ("error out"=w818:errorcluster, "Data Out"=w822:T8, "LoadSensors"=w820:dbl[], "Raw Data"=w819:u16[])  [unwired: 6 in]
        n344 = local write "Adj.Data"(w820) -> ()
        n345 = local write "RawData"(w819) -> ()
      }
      frame "Battery Test" {
        # "Final Test>>move to end of test"
        n346 = call "Batt Test.vi"("Error In"=w828, "Data Cluster in"=w829) -> ("Error Out"=w826:errorcluster, "Data Cluster out"=w825:T8)  [unwired: 8 in]
      }
      frame "------RESULTS-------" {
        # "USED ONLY AS HEADER"
      }
      frame "End Test" {
        n347 = Unbundle By Name(w834) -> ("Cal Retry?"=w833:bool)
        n348 = case shown="참" w833 {
          tunnel: w845 -> [w852 w856]
          tunnel: [w851 w856] -> w844
          frame False {
            n349 = property on="CaptureButton" class="Bool (엄격한)"(error in=w852, "Visible"=FALSE, "DisabledEnum"=T21."Disabled" ("Disabled"), "Value"=FALSE ("CaptureButton")) -> (error out=w851:errorcluster)  [unwired: 1 in, 1 out]
          }
          frame True {
          }
        }
        n350 = call "Store Results.vi"("error in (no error)"=w844, "Data In"=w834) -> ("error out"=w848:errorcluster, "Data Out"=w847:T8)  [unwired: 8 in]
        n351 = control-ref of="Test Result"() -> (w850:refnum<vi>)
        n352 = call "Failed Test Logic.vi"("error in (no error)"=w848, "Test Result"=w850, "State-machine Local Variables in"=w847) -> ("error out"=w843:errorcluster, "Data Out"=w842:T8)  [unwired: 7 in]
        n353 = Unbundle By Name(w842) -> ("Cal Retry?"=w838:bool)
        n354 = case shown="참" w838 {
          frame False {
            w859 = T21."Enabled" ("Disabled")
            n355 = local write "Target Serial#:"(u32 0 ("Serial#:")) -> ()
            n356 = property on="Message" class="Str"("Blinking"=FALSE) -> ()  [unwired: 2 in, 2 out]
            n357 = property on="Correction Factor" class="Str"("DisabledEnum"=w859) -> ()  [unwired: 2 in, 2 out]
            n358 = property on="Target Serial#:" class="DigNum (엄격한)"("DisabledEnum"=w859) -> ()  [unwired: 2 in, 2 out]
            n359 = property on="Shutdown Dev" class="Bool"("DisabledEnum"=w859) -> ()  [unwired: 2 in, 2 out]
            n360 = property on="Scan Channels" class="Bool"("DisabledEnum"=w859) -> ()  [unwired: 2 in, 2 out]
            n361 = property on="Operating Channel" class="CmbBox"("DisabledEnum"=w859) -> ()  [unwired: 2 in, 2 out]
            n362 = property on="Start Channel" class="CmbBox (엄격한)"("DisabledEnum"=w859) -> ()  [unwired: 2 in, 2 out]
          }
          frame True {
          }
        }
        n363 = Select(t=TRUE ("Serial Table.Valid Serial?"), s=w838, f=FALSE ("Serial Table.Valid Serial?")) -> (s? t:f=w835:bool)
        n364 = Select(t=Gen2_FT_states."Load Test" ("NextState"), s=w838, f=Gen2_FT_states."Shutdown Device" ("NextState")) -> (s? t:f=w839:T6)
        n365 = Bundle By Name(cluster=w842, "Serial Table.Valid Serial?"=w835, "NextState"=w839) -> (w849:T8)
      }
      frame "Display Result" {
        n366 = call "RxBuffer.vi"("error in (no error)"=w892) -> ("DeviceParameters"=w863:T29, "LoadSensors"=w873:dbl[], "RxData Out"=w861:u16[], "DUT Serial Number"=→"Streaming Serial Number":u32, "New Data"=w874:bool, "error out"=w891:errorcluster)  [unwired: 7 in, 6 out]
        n367 = Unbundle By Name(w863) -> ("GotCal"=→"GotCal":bool)
        n368 = local write "Adj.Data"(w873) -> ()
        n369 = Unbundle By Name(w870) -> ("DUT Parameters.Batt310"=w869:u16, "DUT Parameters.Batt 280"=w868:u16, "DUT Parameters"=→"Device Parameters":T3)
        n370 = Unbundle By Name(w870) -> ("Message"=w876:string)
        n371 = call "BatchTest HeartBeat.vi"("MaxTime"=u32 3000, "Value In"=w874) -> ("Alive?"=w888:bool)  [unwired: 8 in, 1 out]
        n372 = Array Subset(array=w861, index=2) -> (→"RawData":u16[])  [unwired: 1 in]
        n373 = call "Mark10.vi"("Data In"=w870, "error in (no error)"=w891, "Action"=Mark10_states."Read Status") -> ("Live Load"=w883:dbl, "Live Position"=w880:dbl, "error out"=w877:errorcluster)  [unwired: 12 in, 2 out]
        n374 = Index Array(array=w861, index=10) -> (element=w871:u16)
        n375 = call "BatchTest BoolValue Change.vi"("Value In"=w888) -> ("Value Changed?"=w890:bool, "Value Out"=w889:bool)  [unwired: 7 in, 2 out]
        n376 = First Call?() -> (First Call?: T/F=w885:bool)
        n377 = Or(x=w890, y=w885) -> (x .or. y?=w886:bool)
        n378 = case shown="에러 없음" w877 {
          selector: w877 -> [w895 _]
          tunnel: w883 -> [w897 w900]
          tunnel: [w897 w900] -> w882
          tunnel: [w896 w899] -> w881
          tunnel: w880 -> [w896 w899]
          tunnel: [w895 errorcluster {"status"=FALSE, "code"=0, "source"=""} ("error IO")] -> w879
          tunnel: [w894 "Issue with Mark-10.\nMake sure unit is on and \ntry again. " ("Message")] -> w878
          tunnel: w876 -> [w894 _]
          frame No Error {
          }
          frame Error {
          }
        }
        n379 = case shown="참" w886 {
          tunnel: w889 -> [_ w903]
          frame False {
          }
          frame True {
            n380 = local read "Test Device"() -> (w904:bool)
            n381 = And(x=w903, y=w904) -> (x .and. y?=w902:bool)
            n382 = case shown="거짓" w902 {
              tunnel: w903 -> [w905 w906]
              frame False {
                # "Can Trigger Value Signaling"
                # "Device is OFF or Test is OFF"
                n383 = property on="Device ON?" class="Bool (엄격한)"("Val(Sgnl)"=w905) -> ()  [unwired: 2 in, 2 out]
              }
              frame True {
                # "Can turn on LED only"
                # "Test is ON AND Device is ON"
                n384 = local write "Device ON?"(w906) -> ()
              }
            }
          }
        }
        n385 = call "Calc Battery.vi"("Batt 280"=w868, "Batt310"=w869, "AD"=w871) -> ("Batt Volt"=→"Battery Voltage":dbl)  [unwired: 8 in]
        n386 = Bundle By Name(cluster=w870, "G.Load"=w882, "G.Position"=w881, "Message"=w878) -> (w893:T8)
      }
      frame "--------EXIT--------" {
        # "USED ONLY AS HEADER"
      }
      frame "Exit" {
        n387 = call "Mark10.vi"("Data In"=w912, "error in (no error)"=w914, "Action"=Mark10_states."Stop Motor") -> ("error out"=w917:errorcluster)  [unwired: 12 in, 4 out]
        n388 = call "Mark10.vi"("Data In"=w912, "error in (no error)"=w917, "Action"=Mark10_states."Go Home") -> ("error out"=w915:errorcluster)  [unwired: 12 in, 4 out]
        n389 = call <vilib>:"Clear Errors.vi"("error in (no error)"=w915) -> ("error out"=w913:errorcluster)  [unwired: 5 in, 1 out]
        n390 = First Call?() -> (First Call?: T/F=w925:bool)
        n391 = case shown="참" w925 {
          tunnel: w913 -> [w928 w931]
          tunnel: [w928 w930] -> w923
          tunnel: w912 -> [_ w929]
          frame False {
          }
          frame True {
            n392 = call "Mark10.vi"("Data In"=w929, "error in (no error)"=w931, "Action"=Mark10_states."Exit") -> ("error out"=w930:errorcluster)  [unwired: 12 in, 4 out]
          }
        }
        n393 = local read "Device ON?"() -> (w919:bool)
        n394 = call "Shutdown DUT.vi"("error in (no error)"=w923, "Device On?"=w919, "Blast?"=FALSE, "Data In"=w912) -> ("error out"=w921:errorcluster, "State-machine Local Variables out"=w922:T8)  [unwired: 6 in]
        n395 = flat-sequence {
          tunnel: w921 -> [w927]
          tunnel: [w927] -> w920
          frame #0 {
            n396 = local write "Close Xsceiver"(TRUE ("Close Xsceiver")) -> ()
          }
        }
      }
    }
    n397 = call <vilib>:"Clear Errors.vi"("error in (no error)"=w32) -> ("error out"=w27:errorcluster)  [unwired: 5 in, 1 out]
    "Main" <- w29
  }
  n398 = Wait on Occurrence(2:w19, 3:35000 ("ms timeout (-1)")) -> (0:w5:bool)  [unwired: 1 in]
  n399 = while {
    shift-right: [w939] -> w2
    shift-left: w4 -> [w937]
    tunnel: ["Close Xsceiver"] -> w16
    tunnel: w5 -> [_]
    i -> [w933]
    stop <- "Close Xsceiver" stop-if-true
    n400 = global read "Gen2 FT Globals.vi" "RawRxTx"() -> (w938:bool)
    n401 = call <vilib>:"Clear Errors.vi"("error in (no error)"=w937) -> ("error out"=w936:errorcluster)  [unwired: 5 in, 1 out]
    n402 = case shown="거짓" w938 {
      tunnel: w936 -> [w941 w952]
      tunnel: [w940 w952] -> w939
      frame False {
        n403 = case shown="거짓" "ClearBuffer" {
          tunnel: w941 -> [w946 w949]
          tunnel: [w946 w948] -> w943
          frame False {
            n404 = Wait Until Next ms Multiple(millisecond multiple=u32 5) -> ()  [unwired: 1 out]
          }
          frame True {
            n405 = local write "ClearBuffer"(FALSE ("ClearBuffer")) -> ()
            n406 = call "RxTx.vi"("error in (no error)"=w949, "Action"=XceiverStates."Clear Buffer") -> ("error out"=w948:errorcluster)  [unwired: 9 in, 8 out]
          }
        }
        n407 = call "RxTx.vi"("error in (no error)"=w943, "Action"=XceiverStates."Rx") -> ("error out"=w940:errorcluster)  [unwired: 9 in, 8 out]
      }
      frame True {
        n408 = Wait Until Next ms Multiple(millisecond multiple=u32 100) -> ()  [unwired: 1 out]
      }
    }
    n409 = Get Date/Time In Seconds() -> (seconds since 1Jan1904=→"Current Time:":timestamp)
    "Read" <- w933
  }
  n410 = case shown="거짓" w16 {
    frame False {
      n411 = property on="Exit" class="Bool"("Val(Sgnl)"=TRUE ("Value (Signaling)")) -> ()  [unwired: 2 in, 2 out]
    }
    frame True {
    }
  }
  n412 = call <vilib>:"Clear Errors.vi"("error in (no error)"=w2) -> ("error out"=w1:errorcluster)  [unwired: 5 in, 1 out]
  n413 = call "RxTx.vi"("error in (no error)"=w1, "Action"=XceiverStates."Close") -> ("error out"=w17:errorcluster)  [unwired: 9 in, 8 out]
  n414 = local write "Close Xsceiver"(w7) -> ()
  n415 = Merge Errors(w17, w20) -> (w15:errorcluster)
  n416 = call <vilib>:"Clear Errors.vi"("error in (no error)"=w15) -> ("error out"=w13:errorcluster)  [unwired: 5 in, 1 out]
  n417 = call <vilib>:"Simple Error Handler.vi"("type of dialog (OK msg:1)"=w14, "error in (no error)"=w13) -> ("error out"=w12:errorcluster)  [unwired: 3 in, 4 out]
  n418 = disable-structure shown="RUN_TIME_ENGINE==True" {
    disable-tunnel: w12 -> [w954 w955]
    disable-tunnel: [w954 w955] -> w11
    frame condition #0 {
      n419 = Quit LabVIEW() -> ()  [unwired: 1 in]
    }
    frame condition #1 (active) {
    }
  }
  "error out" <- w11
